vi "Laser.vi"() -> ()   [LabVIEW 2013]
doc: "Пограмма управления мишенью лазерного источника ионов."
uses:
  <vilib>/Utility/miscctls.llb/LVPositionTypeDef.ctl
  <vilib>/Utility/inputDevices.llb/closeJoystick.vi
  <vilib>/Utility/inputDevices.llb/mouseAcquire.vi
panel:
  out "prog ON":string
  out "on event":string
  out "send string":string
  in  "выстрел Y дейт":u16 step=1
  out "Статус":bool=TRUE caption="Готов!"
  in  "Параметры М1":T1={"TipStrip"="Мишень 1", "Left"=1, "Top"=1, "Width"=10, "Height"=10, "Шаг перехода по горизонтали"=3, "Шаг перехода по горизонтали"=3, "Выстрелов до перехода"=10}
  out "Знак Графит Dx":i8=100
  out "Знак LiF2 Dx":i8=100
  out "Знак LiF1 Dx":i8=100
  out "Знак дейт Dx":i8=100
  in  "выстрел  Y Графит":u16 step=1
  in  "выстрел X Графит":u16 step=1
  in  "выстрел Y LiF 2":u16 step=1
  in  "выстрел X LiF 2":u16 step=1
  in  "выстрел Y LiF 1":u16 step=1
  in  "выстрел X LiF 1":u16 step=1
  in  "выстрел X дейт":u16 step=1
  in  "xxx":enum32{" Мишени", " Настройки TCP"}(tab)
  in  "XY лазера":bool
  in  "LiF 1":picture
  in  "Звук выстрела":bool
  in  "Мишень 2":picture
  in  "Мишень 1":picture
  in  "OK Button":bool
  in  "Графит":picture
  in  "Дейтерий":picture
  in  "Выстрелов до перемотки":u16=100
  in  "id мишени":u16=1
  in  "Счетчик выстрелов:":u32
  in  "Шаг перехода по Y графит":dbl=1.0 format="%.1f"
  in  "Шаг перехода по Х графит":dbl=1.0 format="%.1f"
  in  "Выстрелов в точку  графит":u16=3
  in  "Шаг перехода по Y LiF 2":dbl=1.0 format="%.1f"
  in  "Шаг перехода по Х LiF 2":dbl=1.0 format="%.1f"
  in  "Выстрелов в точку  LiF 2":u16=3
  in  "Шаг перехода по Y LiF 1":dbl=1.0 format="%.1f"
  in  "Шаг перехода по Х LiF 1":dbl=1.0 format="%.1f"
  in  "Выстрелов в точку LiF 1":u16=3
  in  "Шаг перехода по Y дейт":dbl=1.0 min=0.0 format="%.1f"
  in  "Шаг перехода по Х дейт":dbl=1.0 min=0.0 format="%.1f"
  in  "Выстрелов в точку дейтерий":u16=3
  in  "TCP read data":string
  in  "LiF 2":picture
  out "Slide X axis":u8(slide) max=100 scale=0.0..100.0
  out "Slide Y axis":u8(slide) max=50 step=1
  in  "Снимок":bool
  out "con err":bool caption="Connect"
  out "Con":bool
  out "Mouse on Pane pos Horizontal":i32
  out "Mouse on Pane pos Vertical":i32
  in  "Выстрел по мишени!":u32
  out "Выбор миш 1":bool
  out "Выбор миш 2":bool
  out "Выбор миш 3":bool
  out "Выбор миш 4":bool
  out "Счетчик мишеней":u16=3
  out "Шаг перехода по горизонтали":u16
  out "Шаг перехода по вертикали":u16
  out "Выстрелов до перехода":u16
  in  "порт":u16=10001
  in  "IP-адрес":string="159.93.126.157"
  in  "Disconnect":bool caption="Disconn"
  out "Connected":bool
  in  "Connect":bool
  out "TCP error source":string
  in  "stop":bool
  out "read_error_indicator":bool
  in  "Connect 2":bool caption="Connect"
  in  "flag1":bool caption="Disconn"
  out "x+1":dbl
  out "TCP con ID":refnum<k5>
  # "LiF 1"
  # "Дейтерированный полиэтилен"
  # "LiF 2"
  # "Графит"
  # "LiF 1"
  # "Графит"
  # "Дейтерированный полиэтилен"
  # "Шаг перехода по Y, мм"
  # "Шаг перехода по Х, мм"
  # "Выстрелов в точку"
  # "Выстрелов в точку"
  # "Шаг перехода по Х, мм"
  # "Шаг перехода по Y, мм"
  # "Выстрелов в точку"
  # "Шаг перехода по Х, мм"
  # "Шаг перехода по Y, мм"
  # "Выстрелов в точку"
  # "Шаг перехода по Х, мм"
  # "Шаг перехода по Y, мм"
  # "LiF 2"
types:
  T1 = cluster{"TipStrip":string, "Left":i32, "Top":i32, "Width":u16, "Height":u16, "Шаг перехода по горизонтали":u16, "Шаг перехода по горизонтали":u16, "Выстрелов до перехода":u16}
  T2 = typedef "LVPositionTypeDef.ctl" = cluster{"Left":i32, "Top":i32}
  T3 = enum8{"Enabled", "Disabled", "Disabled and Grayed Out"}
  T4 = typedef "imagedata.ctl" = cluster{"image type":i32, "image depth":i32, "image":u8[], "mask":u8[], "colors":u32[], "Rectangle":cluster{"left":i16, "top":i16, "right":i16, "bottom":i16}}
  T5 = typedef "LVRectTypeDef.ctl" = cluster{"Left":i16, "Top":i16, "Right":i16, "Bottom":i16}
  T6 = cluster{"Horizontal":i32, "Vertical":i32, "Scrolling":i32}
  T7 = cluster{"Название мишени":string, "Х0":u16, "Y0":u16, "Длина, мм":u16, "Ширина, мм":u16, "Шаг перехода по горизонтали":u16, "Шаг перехода по вертикали":u16, "Выстрелов до перехода":u16}
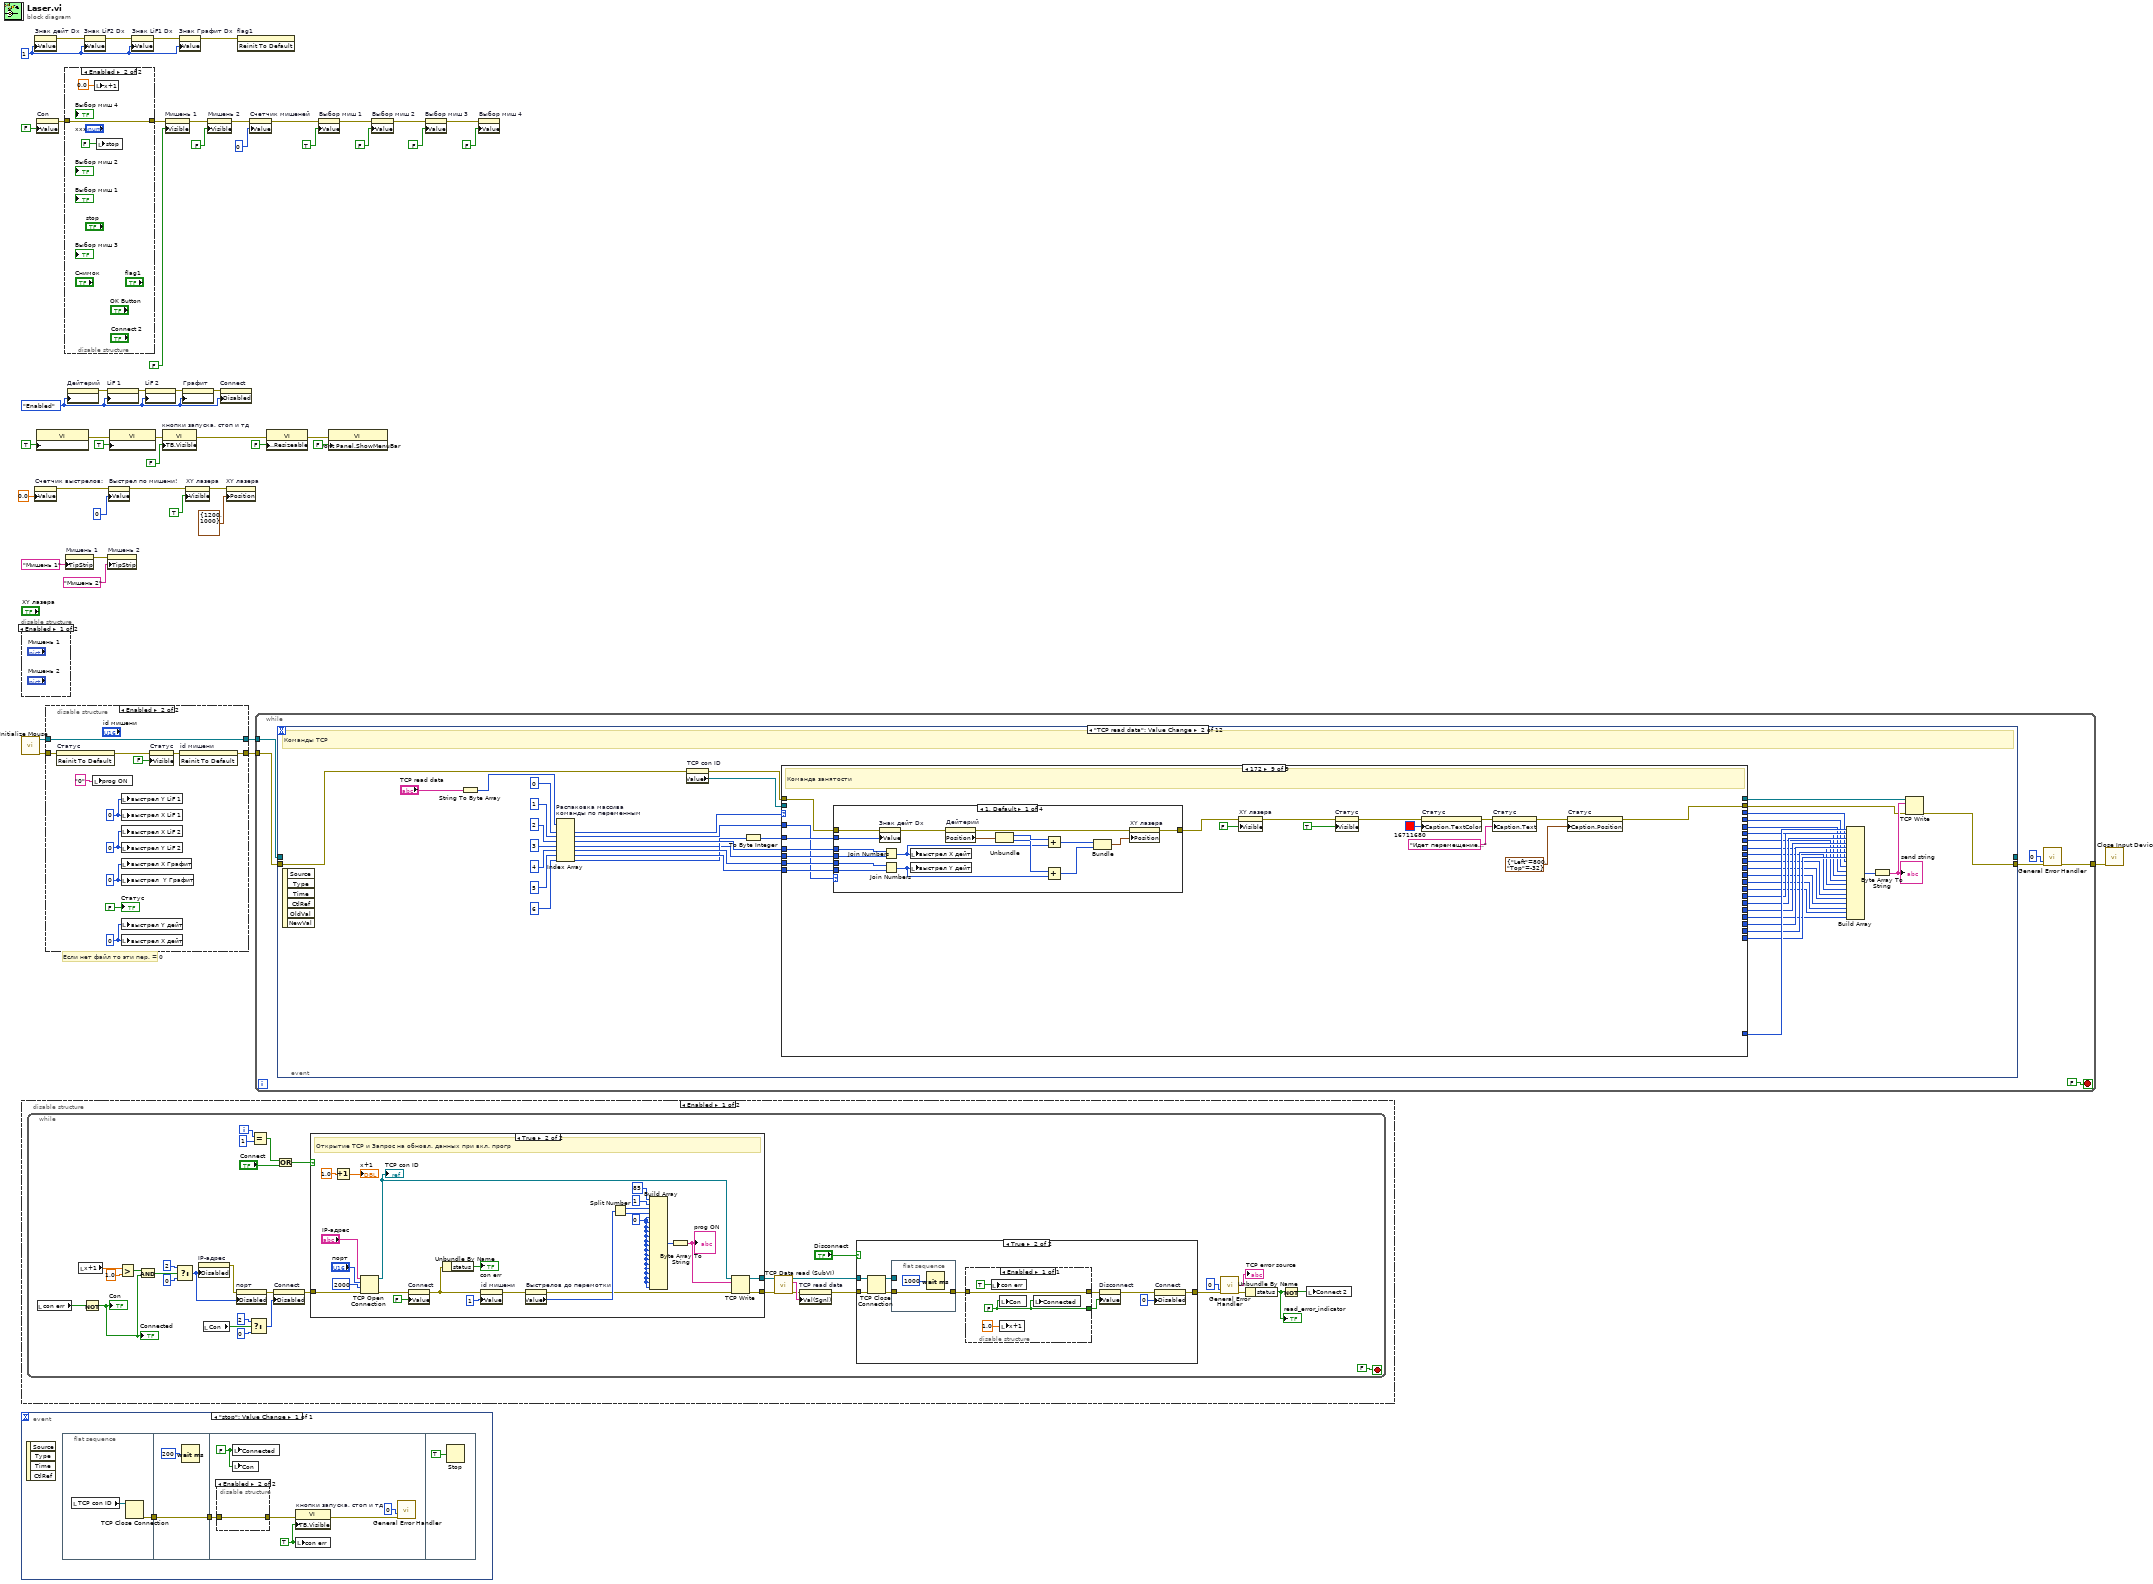
[diagram p0: block diagram]
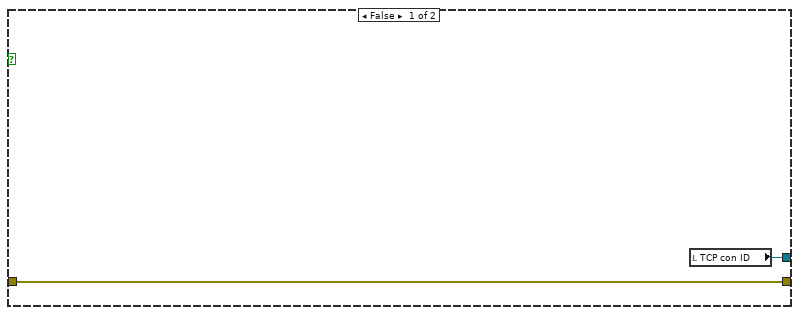
[diagram p3: hidden frame]
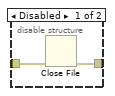
[diagram p8: hidden frame]
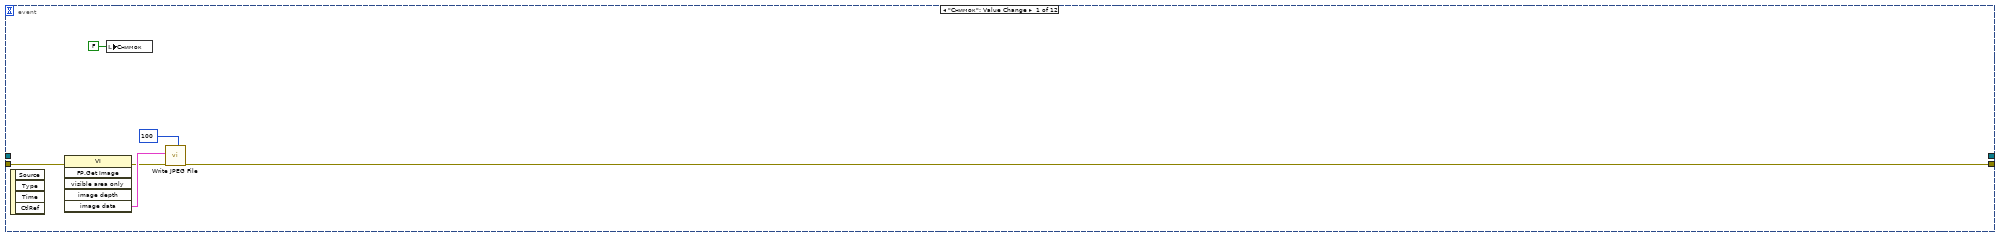
[diagram p9: hidden frame]
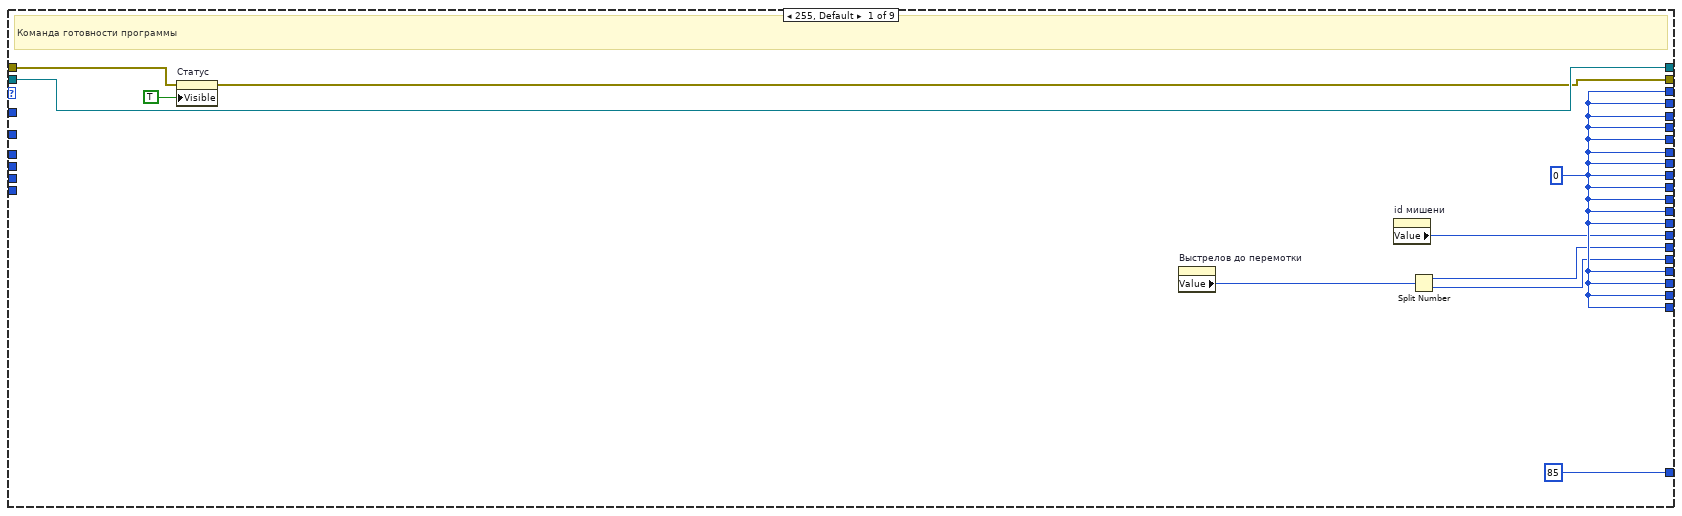
[diagram p10: hidden frame]
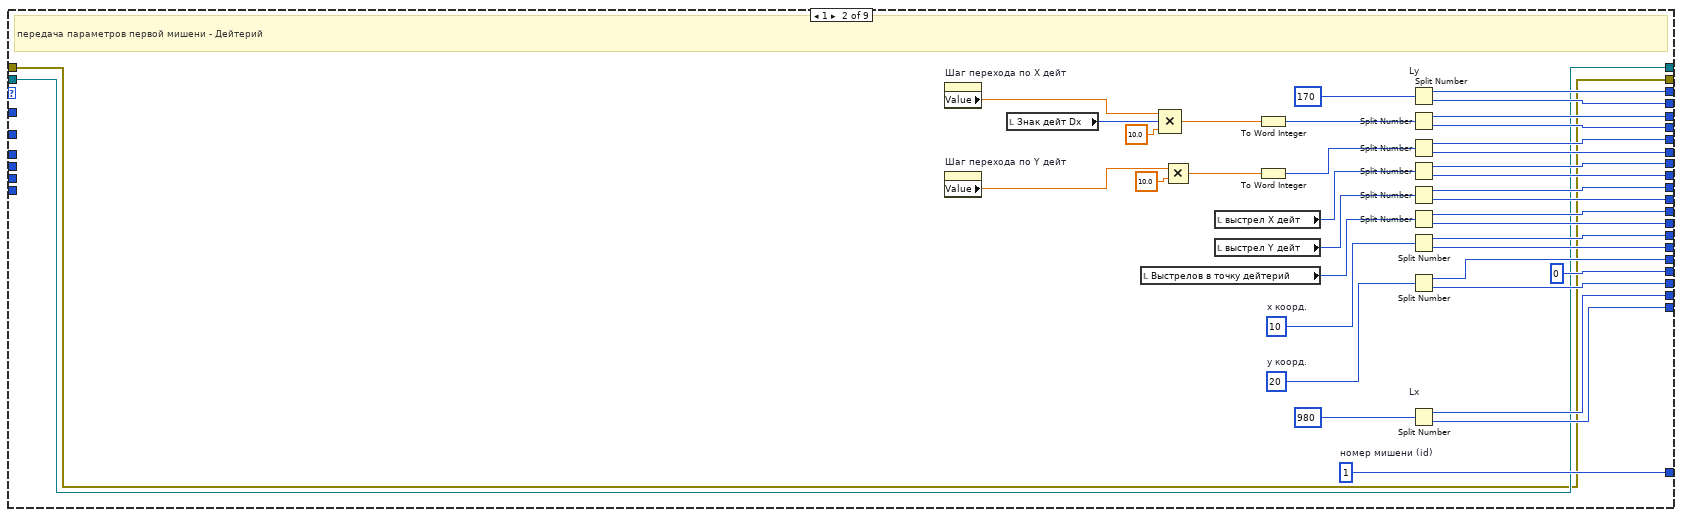
[diagram p11: hidden frame]
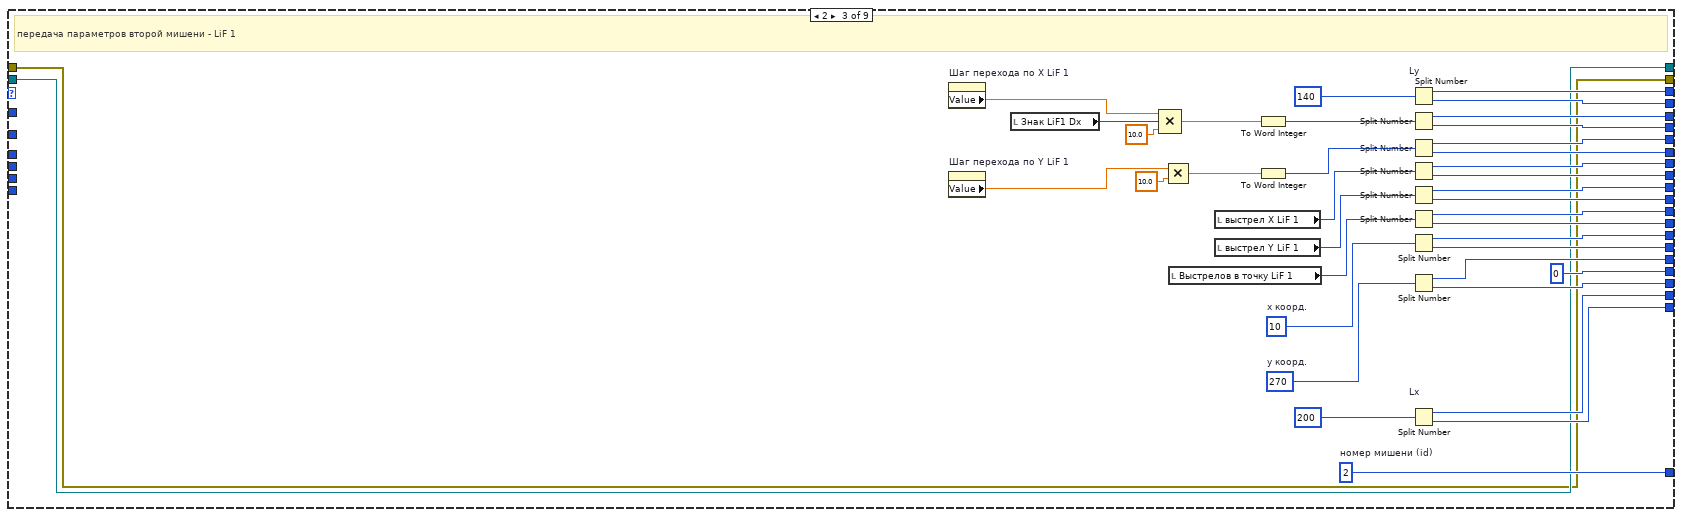
[diagram p12: hidden frame]
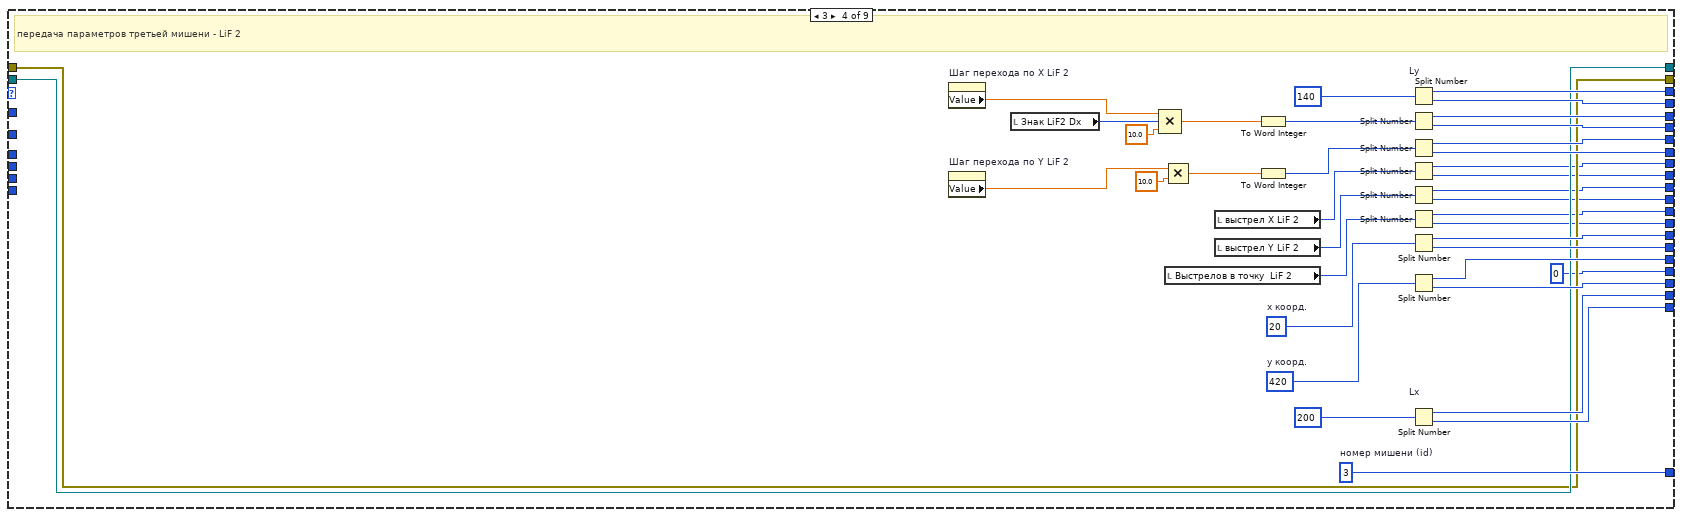
[diagram p13: hidden frame]
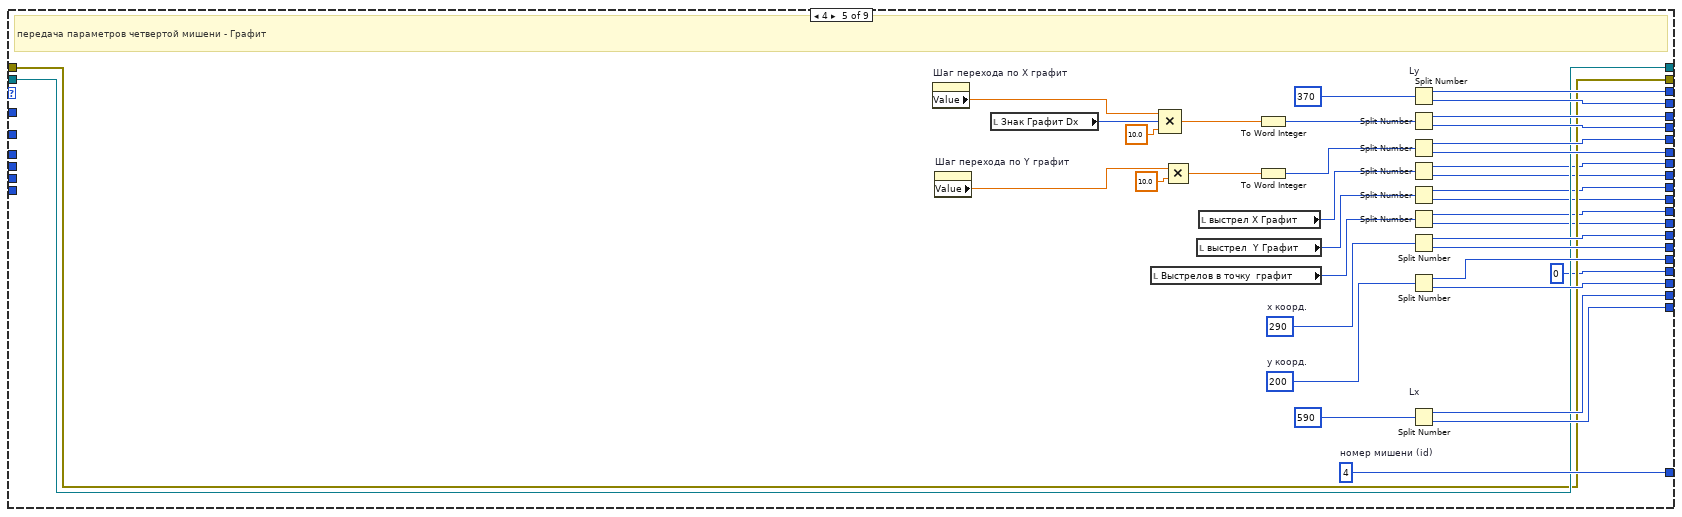
[diagram p14: hidden frame]
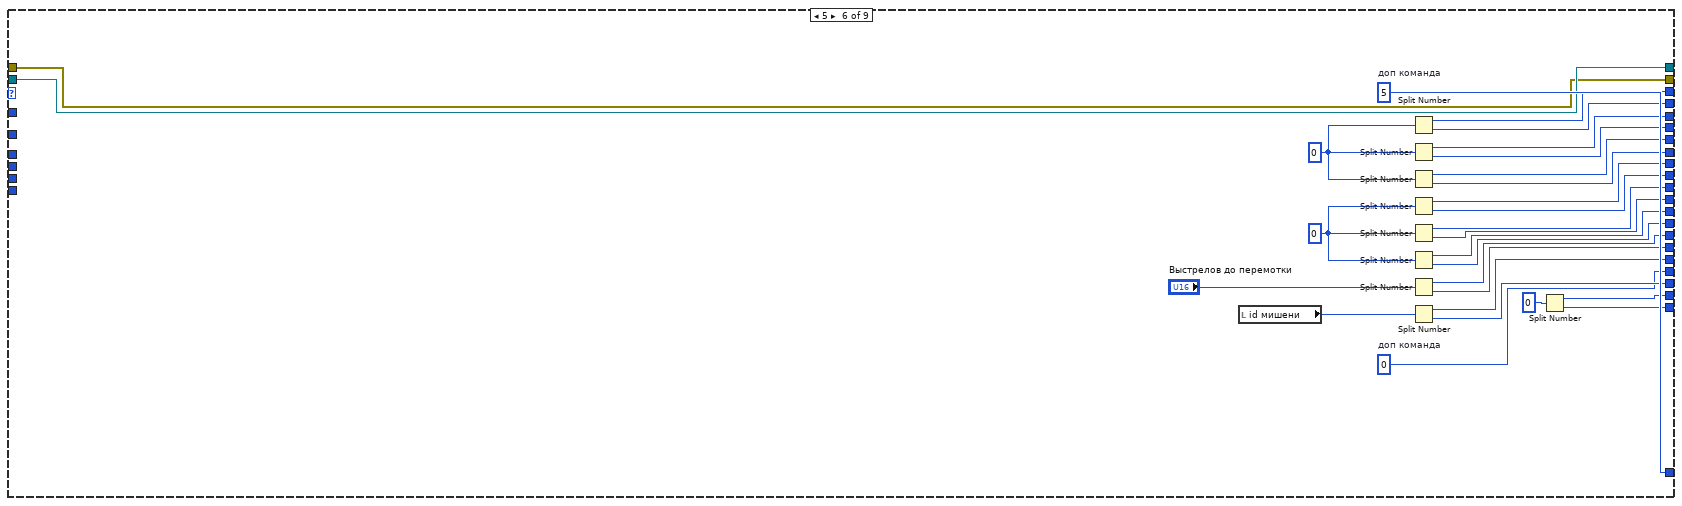
[diagram p15: hidden frame]
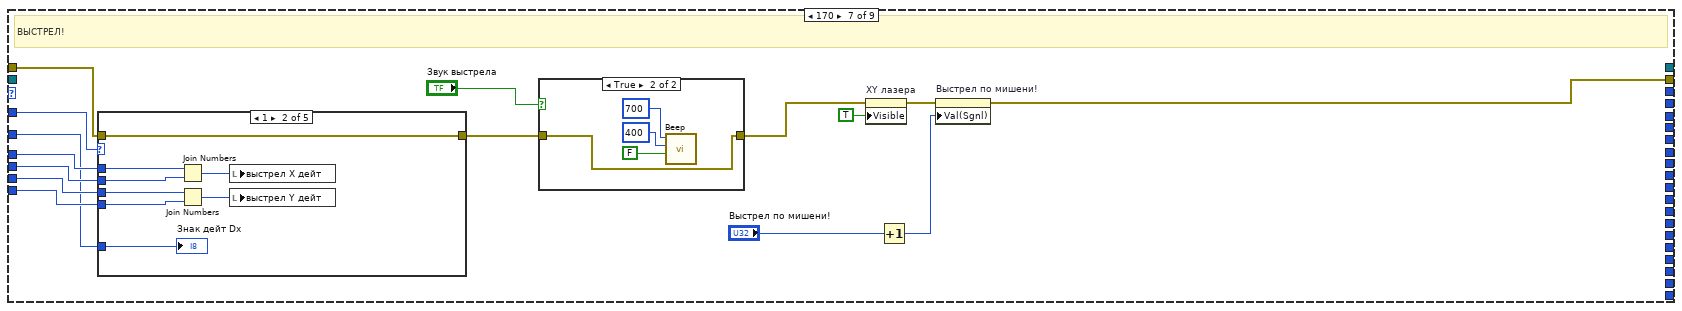
[diagram p16: hidden frame]
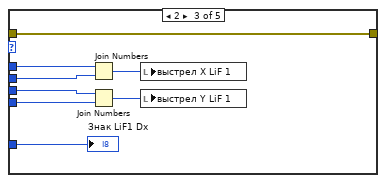
[diagram p19: hidden frame]
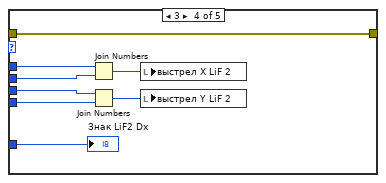
[diagram p20: hidden frame]
diagram:
  w16 = i8 1 ("Знак дейт Dx")
  w2 = T3."Enabled" ("Disabled")
  # "Если нет файл то эти пер. = 0"
  n1 = disable-structure shown="Enabled" {
    frame Enabled {
    }
    frame Disabled {
    }
  }
  n2 = call <vilib>:"Initialize Mouse.vi"() -> ("error out"=w9:errorcluster, "device ID"=w11:refnum<k1>)  [unwired: 1 in, 9 out]
  n3 = disable-structure shown="Enabled" {
    frame Enabled {
      n4 = while {
        i -> [w77]
        stop <- FALSE stop-if-true
        n5 = local read "con err"() -> (w65:bool)
        n6 = local read "x+1"() -> (w68:dbl)
        n7 = Not(x=w65) -> (.not. x?=w64:bool)
        "Connected" <- w64
        "Con" <- w64
        n8 = Greater?(x=w68, y=1.0) -> (0:w66:bool)
        n9 = And(x=w66, y=w64) -> (x .and. y?=w61:bool)
        n10 = Select(t=u8 2 ("Disabled"), s=w61, f=u8 0 ("Disabled")) -> (s? t:f=w83:u8)
        n11 = property on="IP-адрес" class="Str"("Disabled"=w83) -> (error out=w82:errorcluster)  [unwired: 2 in, 1 out]
        n12 = local read "Con"() -> (w58:bool)
        n13 = property on="порт" class="DigNum (strict)"(error in=w82, "Disabled"=w83) -> (error out=w81:errorcluster)  [unwired: 1 in, 1 out]
        n14 = Select(t=u8 2 ("Disabled"), s=w58, f=u8 0 ("Disabled")) -> (s? t:f=w70:u8)
        n15 = Equal?(x=w77, y=1) -> (x = y?=w78:bool)
        n16 = property on="Connect" class="Bool (strict)"(error in=w81, "Disabled"=w70) -> (error out=w75:errorcluster)  [unwired: 1 in, 1 out]
        n17 = Or(x=w78, y="Connect") -> (x .or. y?=w80:bool)
        n18 = case shown="True" w80 {
          tunnel: [w87 w91] -> w55
          tunnel: w75 -> [w87 w103]
          tunnel: [w86 w90] -> w54
          frame False {
            n19 = local read "TCP con ID"() -> (w86:refnum<k5>)
          }
          frame True {
            w98 = u8 0 ("element")
            # "Открытие TCP и Запрос на обновл. данных при вкл. прогр"
            n20 = Increment(x=1.0) -> (x+1=→"x+1":dbl)
            n21 = TCP Open Connection(address="IP-адрес", remote port or service name="порт", timeout ms (60000)=2000, error in (no error)=w103) -> (connection ID=w88:refnum<k5>, error out=w105:errorcluster)  [unwired: 1 out]
            "TCP con ID" <- w88
            n22 = property on="Connect" class="Bool (strict)"(error in=w105, "Value"=FALSE ("Connect")) -> (error out=w93:errorcluster)  [unwired: 1 in, 1 out]
            n23 = Unbundle By Name(w93) -> ("status"=→"con err":bool)
            n24 = property on="id мишени" class="DigNum (strict)"(error in=w93, "Value"=u16 1 ("id мишени")) -> (error out=w95:errorcluster)  [unwired: 1 in, 1 out]
            n25 = property on="Выстрелов до перемотки" class="DigNum (strict)"(error in=w95) -> (error out=w92:errorcluster, "Value"=w99:u16)  [unwired: 1 in, 1 out]
            n26 = Split Number(x=w99) -> (hi(x)=w97:u8, lo(x)=w96:u8)
            n27 = Build Array(u8 85 ("element"), u16 1 ("id мишени"), w97, w96, w98, w98, w98, w98, w98, w98, w98, w98, w98, w98, w98, w98, w98, w98, w98, w98) -> (w101:u16[])
            n28 = Byte Array To String(unsigned byte array=w101) -> (string=w100:string)
            "prog ON" <- w100
            n29 = TCP Write(connection ID=w88, data in=w100, error in (no error)=w92) -> (connection ID out=w90:refnum<k5>, error out=w91:errorcluster)  [unwired: 1 in, 1 out]
          }
        }
        n30 = call "TCP Data read (SubVI).vi"("error in (no error)"=w55, "TCP Network Connection in"=w54) -> ("error out"=w56:errorcluster, "Read data"=w71:string, "TCP Network Connection out"=w73:refnum<k5>)  [unwired: 1 in, 6 out]
        n31 = property on="TCP read data" class="Str"(error in=w56, "Val(Sgnl)"=w71) -> (error out=w57:errorcluster)  [unwired: 1 in, 1 out]
        n32 = case shown="True" "Disconnect" {
          tunnel: [w112 w118] -> w52
          tunnel: w57 -> [w112 w117]
          tunnel: w73 -> [_ w116]
          frame False {
          }
          frame True {
            n33 = TCP Close Connection(connection ID=w116, error in (no error)=w117) -> (connection ID out=w120:refnum<k5>, error out=w119:errorcluster)  [unwired: 1 out]
            n34 = flat-sequence {
              tunnel: w120 -> [_]
              tunnel: w119 -> [w127]
              tunnel: [w127] -> w113
              frame #0 {
                n35 = Wait (ms)(milliseconds to wait=u32 1000) -> ()  [unwired: 1 out]
              }
            }
            n36 = disable-structure shown="Enabled" {
              disable-tunnel: [w124] -> w115
              disable-tunnel: [w123] -> w114
              disable-tunnel: w113 -> [w123]
              frame Enabled {
                w124 = FALSE ("Disconnect")
                n37 = local write "con err"(TRUE ("con err")) -> ()
                n38 = local write "Con"(w124) -> ()
                n39 = local write "x+1"(1.0 ("1")) -> ()
                n40 = local write "Connected"(w124) -> ()
              }
            }
            n41 = property on="Disconnect" class="Bool (strict)"(error in=w114, "Value"=w115) -> (error out=w121:errorcluster)  [unwired: 1 in, 1 out]
            n42 = property on="Connect" class="Bool (strict)"(error in=w121, "Disabled"=u8 0) -> (error out=w118:errorcluster)  [unwired: 1 in, 1 out]
          }
        }
        n43 = call <vilib>:"General Error Handler.vi"("type of dialog (OK msg:1)"=u8 0, "error in (no error)"=w52) -> ("source out"=→"TCP error source":string, "error out"=w51:errorcluster)  [unwired: 12 out]
        n44 = Unbundle By Name(w51) -> ("status"=w53:bool)
        "read_error_indicator" <- w53
        n45 = Not(x=w53) -> (.not. x?=w85:bool)
        n46 = local write "Connect 2"(w85) -> ()
      }
    }
    frame Disabled {
    }
  }
  n47 = event shown="[0] \"stop\": Value Change" {
    selector: _ -> [_]
    dyn-events: _ -> [_]
    timeout: _ -> [_]
    event "stop": Value Change {
      n48 = event-data() -> ()  [unwired: 5 out]
      n49 = flat-sequence {
        tunnel: [w131] -> w130
        tunnel: w130 -> [w134]
        tunnel: [w134] -> w129
        tunnel: w129 -> [w138]
        frame #0 {
          n50 = local read "TCP con ID"() -> (w132:refnum<k5>)
          n51 = TCP Close Connection(connection ID=w132) -> (error out=w131:errorcluster)  [unwired: 1 in, 2 out]
        }
        frame #1 {
          n52 = Wait (ms)(milliseconds to wait=u32 200) -> ()  [unwired: 1 out]
        }
        frame #2 {
          w140 = FALSE ("Запись в файл")
          w139 = TRUE ("Tool Bar:Visible")
          n53 = disable-structure shown="Enabled" {
            disable-tunnel: [w142 w143] -> w136
            disable-tunnel: w138 -> [w141 w143]
            frame Disabled {
              n54 = Close File(error in=w141) -> (error out=w142:errorcluster)  [unwired: 1 in, 1 out]
            }
            frame Enabled {
            }
          }
          n55 = local write "Connected"(w140) -> ()
          n56 = local write "Con"(w140) -> ()
          n57 = property on="кнопки запуска, стоп и тд" class="VI"(error in=w136, "TB.Visible"=w139) -> (error out=w137:errorcluster)  [unwired: 1 in, 1 out]
          n58 = local write "con err"(w139) -> ()
          n59 = call <vilib>:"General Error Handler.vi"("type of dialog (OK msg:1)"=u32 0 ("milliseconds to wait"), "error in (no error)"=w137) -> ()  [unwired: 14 out]
        }
        frame #3 {
          n60 = Stop(stop? (T)=TRUE) -> ()
        }
      }
    }
  }
  n61 = property on="Знак дейт Dx" class="DigNum (strict)"("Value"=w16) -> (error out=w15:errorcluster)  [unwired: 2 in, 1 out]
  n62 = property on="Счетчик выстрелов:" class="DigNum (strict)"("Value"=0.0 ("Счетчик выстрелов:")) -> (error out=w32:errorcluster)  [unwired: 2 in, 1 out]
  n63 = property on="Con" class="Bool (strict)"("Value"=FALSE ("Connected")) -> (error out=w38:errorcluster)  [unwired: 2 in, 1 out]
  n64 = property class="VI"("Front Panel.Minimizeable"=TRUE ("Front Panel Window:Minimizable")) -> (error out=w44:errorcluster)  [unwired: 2 in, 1 out]
  n65 = disable-structure shown="Enabled" {
    disable-tunnel: [_ w152] -> w12
    disable-tunnel: w11 -> [_ w152]
    disable-tunnel: [_ w147] -> w10
    disable-tunnel: w9 -> [_ w150]
    frame Disabled {
    }
    frame Enabled {
      w153 = u16 0 ("выстрел  Y Графит")
      w154 = u16 0 ("выстрел Y LiF 2")
      w155 = u16 0 ("выстрел X LiF 1")
      w156 = u16 0 ("выстрел X дейт")
      n66 = invoke on="Статус" class="Bool (strict)" method="Reinit To Default"(error in=w150) -> (error out=w148:errorcluster)  [unwired: 2 in, 2 out]
      n67 = local write "prog ON"("0" ("prog ON")) -> ()
      n68 = local write "выстрел Y LiF 1"(w155) -> ()
      n69 = local write "выстрел X LiF 1"(w155) -> ()
      n70 = local write "выстрел X LiF 2"(w154) -> ()
      n71 = local write "выстрел Y LiF 2"(w154) -> ()
      n72 = local write "выстрел X Графит"(w153) -> ()
      n73 = local write "выстрел  Y Графит"(w153) -> ()
      n74 = local write "выстрел Y дейт"(w156) -> ()
      n75 = local write "выстрел X дейт"(w156) -> ()
      n76 = property on="Статус" class="Bool (strict)"(error in=w148, "Visible"=FALSE) -> (error out=w146:errorcluster)  [unwired: 1 in, 1 out]
      n77 = invoke on="id мишени" class="DigNum (strict)" method="Reinit To Default"(error in=w146) -> (error out=w147:errorcluster)  [unwired: 2 in, 2 out]
      "Статус" <- FALSE ("Готов")
    }
  }
  n78 = disable-structure shown="Enabled" {
    disable-tunnel: [_ w157] -> w3
    disable-tunnel: w38 -> [_ w157]
    frame Disabled {
    }
    frame Enabled {
      n79 = local write "x+1"(0.0 ("x+1")) -> ()
      n80 = local write "stop"(FALSE ("Boolean")) -> ()
    }
  }
  n81 = property on="Мишень 1" class="Pict"("TipStrip"="Мишень 1" ("Tip Strip")) -> (error out=w6:errorcluster)  [unwired: 2 in, 1 out]
  n82 = property on="Дейтерий" class="Pict"("DisabledEnum"=w2) -> (error out=w22:errorcluster)  [unwired: 2 in, 1 out]
  n83 = property on="Знак LiF2 Dx" class="DigNum (strict)"(error in=w15, "Value"=w16) -> (error out=w14:errorcluster)  [unwired: 1 in, 1 out]
  n84 = property on="LiF 1" class="Pict"(error in=w22, "DisabledEnum"=w2) -> (error out=w21:errorcluster)  [unwired: 1 in, 1 out]
  n85 = property on="Мишень 2" class="Pict"(error in=w6, "TipStrip"="Мишень 2" ("Tip Strip")) -> ()  [unwired: 1 in, 2 out]
  n86 = property on="Выстрел по мишени!" class="DigNum (strict)"(error in=w32, "Value"=u32 0 ("Выстрел по мишени!")) -> (error out=w19:errorcluster)  [unwired: 1 in, 1 out]
  n87 = property class="VI"(error in=w44, "Front Panel.TitleBarVis"=TRUE ("Front Panel Window:Title Bar Visible")) -> (error out=w43:errorcluster)  [unwired: 1 in, 1 out]
  n88 = property on="Знак LiF1 Dx" class="DigNum (strict)"(error in=w14, "Value"=w16) -> (error out=w13:errorcluster)  [unwired: 1 in, 1 out]
  n89 = property on="LiF 2" class="Pict"(error in=w21, "DisabledEnum"=w2) -> (error out=w20:errorcluster)  [unwired: 1 in, 1 out]
  n90 = property on="кнопки запуска, стоп и тд" class="VI"(error in=w43, "TB.Visible"=FALSE ("Tool Bar:Visible")) -> (error out=w42:errorcluster)  [unwired: 1 in, 1 out]
  n91 = property on="Мишень 1" class="Pict"(error in=w3, "Visible"=FALSE) -> (error out=w36:errorcluster)  [unwired: 1 in, 1 out]
  n92 = property on="Знак Графит Dx" class="DigNum (strict)"(error in=w13, "Value"=w16) -> (error out=w5:errorcluster)  [unwired: 1 in, 1 out]
  n93 = property on="Графит" class="Pict"(error in=w20, "DisabledEnum"=w2) -> (error out=w4:errorcluster)  [unwired: 1 in, 1 out]
  n94 = property on="XY лазера" class="Bool (strict)"(error in=w19, "Visible"=TRUE) -> (error out=w17:errorcluster)  [unwired: 1 in, 1 out]
  n95 = property on="Мишень 2" class="Pict"(error in=w36, "Visible"=FALSE) -> (error out=w33:errorcluster)  [unwired: 1 in, 1 out]
  n96 = property on="Connect" class="Bool (strict)"(error in=w4, "Disabled"=w2) -> ()  [unwired: 1 in, 2 out]
  n97 = property on="XY лазера" class="Bool (strict)"(error in=w17, "Position"=T2 {"Left"=1200, "Top"=1000}) -> ()  [unwired: 1 in, 2 out]
  n98 = invoke on="flag1" class="Bool (strict)" method="Reinit To Default"(error in=w5) -> ()  [unwired: 2 in, 3 out]
  n99 = property on="Счетчик мишеней" class="DigNum (strict)"(error in=w33, "Value"=u16 0 ("Счетчик мишеней")) -> (error out=w24:errorcluster)  [unwired: 1 in, 1 out]
  n100 = while {
    tunnel: w10 -> [w164]
    tunnel: w12 -> [w163]
    tunnel: [w160] -> w1
    stop <- FALSE stop-if-true
    n101 = event shown="[1] \"TCP read data\": Value Change" {
      selector: _ -> [_ _ _ _ _ _ _ _ _ _ _ _]
      dyn-events: _ -> [_ _ _ _ _ _ _ _ _ _ _ _]
      timeout: _ -> [_ _ _ _ _ _ _ _ _ _ _ _]
      tunnel: [w167 w187 w646 w706 w741 w773 w805 w867 w878 w893 w918 _] -> w161
      tunnel: w164 -> [w166 w215 w633 w708 w742 w774 w806 w847 w877 w894 w919 _]
      tunnel: w163 -> [_ _ _ _ _ _ _ w874 _ _ _ _]
      tunnel: [_ _ _ _ _ _ _ w873 _ _ _ _] -> _
      event "Снимок": Value Change {
        n102 = event-data() -> ()  [unwired: 5 out]
        n103 = invoke class="VI" method="FP.Get Image"(error in=w166) -> (error out=w168:errorcluster, "image data"=w169:T4)  [unwired: 5 in, 4 out]
        n104 = local write "Снимок"(FALSE ("Снимок")) -> ()
        n105 = call <vilib>:"Write JPEG File.vi"("quality (80)"=100, "error in (no error)"=w168, "image data"=w169) -> ("error out"=w167:errorcluster)  [unwired: 1 in, 7 out]
      }
      event "TCP read data": Value Change {
        # "Команды TCP"
        n106 = event-data() -> ()  [unwired: 7 out]
        n107 = String To Byte Array(string="TCP read data") -> (unsigned byte array=w180:u8[])
        n108 = Index Array "Распаковка массива\nкоманды по переменным"(array=w180, index #1=0 ("index"), index #2=1 ("index"), index #3=2 ("index"), index #4=3 ("index"), index #5=4 ("index"), index #6=5 ("index"), index #7=6 ("index")) -> (element #1=w212:u8, element #2=w186:u8, element #3=w185:u8, element #4=w172:u8, element #5=w184:u8, element #6=w183:u8, element #7=w182:u8)
        n109 = property on="TCP con ID" class="Ref (strict)"(error in=w215) -> (error out=w214:errorcluster, "Value"=w213:refnum<k5>)  [unwired: 1 in, 1 out]
        n110 = To Byte Integer(number=w182) -> (8bit integer=w181:i8)
        n111 = case shown="172" w212 {
          tunnel: w214 -> [w218 w231 w269 w317 w355 w381 w410 w469 w550]
          tunnel: w213 -> [w225 w232 w270 w318 w356 w392 _ _ _]
          tunnel: [u8 85 ("доп команда") w252 w290 w340 w378 w405 _ _ _] -> w209
          tunnel: [w223 w251 w289 w338 w376 w404 _ _ _] -> w208
          tunnel: [w221 w250 w288 w337 w375 w403 _ _ _] -> w207
          tunnel: [w220 w249 w287 w328 w366 w402 _ _ _] -> w206
          tunnel: [w224 w248 w286 w327 w365 w401 _ _ _] -> w205
          tunnel: [w224 w247 w285 w326 w364 w400 _ _ _] -> w204
          tunnel: [w224 w246 w284 w325 w363 w399 _ _ _] -> w203
          tunnel: [w224 w245 w283 w324 w362 w398 _ _ _] -> w202
          tunnel: [w224 w244 w282 w323 w361 w397 _ _ _] -> w201
          tunnel: [w224 w243 w281 w322 w360 w396 _ _ _] -> w200
          tunnel: [w224 w242 w280 w321 w359 w395 _ _ _] -> w199
          tunnel: [w224 w240 w279 w320 w358 w394 _ _ _] -> w198
          tunnel: [w224 w239 w278 w319 w357 w393 _ _ _] -> w197
          tunnel: [w224 u8 0 u8 0 u8 0 ("номер мишени (id)") u8 0 ("номер мишени (id)") w387 _ _ _] -> w196
          tunnel: [w224 w238 w276 w315 w353 w391 _ _ _] -> w195
          tunnel: [w224 w237 w275 w314 w352 w390 _ _ _] -> w194
          tunnel: [w224 w236 w274 w312 w350 w389 _ _ _] -> w193
          tunnel: [w224 w235 w273 w311 w349 w388 _ _ _] -> w192
          tunnel: [w224 w234 w272 w308 w346 w386 _ _ _] -> w191
          tunnel: [w224 w233 w271 w307 w345 w385 _ _ _] -> w190
          tunnel: [w225 w232 w270 w318 w356 w392 _ _ _] -> w189
          tunnel: [w217 w231 w269 w317 w355 w381 w406 w461 w552] -> w188
          tunnel: w186 -> [_ _ _ _ _ _ w416 w474 w543]
          tunnel: w185 -> [_ _ _ _ _ _ w420 w470 w547]
          tunnel: w172 -> [_ _ _ _ _ _ w419 w471 w546]
          tunnel: w184 -> [_ _ _ _ _ _ w418 w472 w545]
          tunnel: w183 -> [_ _ _ _ _ _ w417 w473 w544]
          tunnel: w181 -> [_ _ _ _ _ _ w411 w465 w548]
          frame 255, Default {
            w224 = u8 0
            # "Команда готовности программы"
            n112 = property on="Статус" class="Bool (strict)"(error in=w218, "Visible"=TRUE) -> (error out=w217:errorcluster)  [unwired: 1 in, 1 out]
            n113 = property on="Выстрелов до перемотки" class="DigNum (strict)"() -> ("Value"=w222:u16)  [unwired: 2 in, 2 out]
            n114 = property on="id мишени" class="DigNum (strict)"() -> ("Value"=w223:u16)  [unwired: 2 in, 2 out]
            n115 = Split Number(x=w222) -> (hi(x)=w221:u8, lo(x)=w220:u8)
          }
          frame 1 {
            w252 = u8 1  # номер мишени (id)
            w260 = u16 20  # y коорд.
            w261 = u16 10  # x коорд.
            # "передача параметров первой мишени - Дейтерий"
            n116 = property on="Шаг перехода по Х дейт" class="DigNum (strict)"() -> ("Value"=w227:dbl)  [unwired: 2 in, 2 out]
            n117 = property on="Шаг перехода по Y дейт" class="DigNum (strict)"() -> ("Value"=w263:dbl)  [unwired: 2 in, 2 out]
            n118 = local read "Знак дейт Dx"() -> (w229:i8)
            n119 = local read "Выстрелов в точку дейтерий"() -> (w253:u16)
            n120 = Compound Arithmetic op=MULTIPLY(w227, w229, 10.0 ("y")) -> (w228:dbl)
            n121 = Multiply(x=w263, y=10.0) -> (x*y=w262:dbl)
            n122 = local read "выстрел X дейт"() -> (w255:u16)
            n123 = local read "выстрел Y дейт"() -> (w254:u16)
            n124 = To Word Integer(number=w228) -> (16bit integer=w257:i16)
            n125 = To Word Integer(number=w262) -> (16bit integer=w256:i16)
            n126 = Split Number "Ly"(x=u16 170) -> (hi(x)=w245:u8, lo(x)=w244:u8)
            n127 = Split Number(x=w257) -> (hi(x)=w243:u8, lo(x)=w242:u8)
            n128 = Split Number(x=w256) -> (hi(x)=w240:u8, lo(x)=w239:u8)
            n129 = Split Number(x=w255) -> (hi(x)=w238:u8, lo(x)=w237:u8)
            n130 = Split Number(x=w254) -> (hi(x)=w236:u8, lo(x)=w235:u8)
            n131 = Split Number(x=w253) -> (hi(x)=w234:u8, lo(x)=w233:u8)
            n132 = Split Number(x=w261) -> (hi(x)=w251:u8, lo(x)=w250:u8)
            n133 = Split Number(x=w260) -> (hi(x)=w249:u8, lo(x)=w248:u8)
            n134 = Split Number "Lx"(x=u16 980) -> (hi(x)=w247:u8, lo(x)=w246:u8)
          }
          frame 2 {
            w290 = u8 2  # номер мишени (id)
            w301 = u16 270  # y коорд.
            w302 = u16 10  # x коорд.
            # "передача параметров второй мишени - LiF 1"
            n135 = property on="Шаг перехода по Х LiF 1" class="DigNum (strict)"() -> ("Value"=w268:dbl)  [unwired: 2 in, 2 out]
            n136 = property on="Шаг перехода по Y LiF 1" class="DigNum (strict)"() -> ("Value"=w296:dbl)  [unwired: 2 in, 2 out]
            n137 = local read "Знак LiF1 Dx"() -> (w265:i8)
            n138 = Compound Arithmetic op=MULTIPLY(w268, w265, 10.0 ("y")) -> (w266:dbl)
            n139 = Multiply(x=w296, y=10.0) -> (x*y=w297:dbl)
            n140 = local read "Выстрелов в точку LiF 1"() -> (w291:u16)
            n141 = local read "выстрел X LiF 1"() -> (w293:u16)
            n142 = local read "выстрел Y LiF 1"() -> (w292:u16)
            n143 = To Word Integer(number=w266) -> (16bit integer=w295:i16)
            n144 = To Word Integer(number=w297) -> (16bit integer=w294:i16)
            n145 = Split Number "Ly"(x=u16 140) -> (hi(x)=w283:u8, lo(x)=w282:u8)
            n146 = Split Number(x=w295) -> (hi(x)=w281:u8, lo(x)=w280:u8)
            n147 = Split Number(x=w294) -> (hi(x)=w279:u8, lo(x)=w278:u8)
            n148 = Split Number(x=w293) -> (hi(x)=w276:u8, lo(x)=w275:u8)
            n149 = Split Number(x=w292) -> (hi(x)=w274:u8, lo(x)=w273:u8)
            n150 = Split Number(x=w291) -> (hi(x)=w272:u8, lo(x)=w271:u8)
            n151 = Split Number(x=w302) -> (hi(x)=w289:u8, lo(x)=w288:u8)
            n152 = Split Number(x=w301) -> (hi(x)=w287:u8, lo(x)=w286:u8)
            n153 = Split Number "Lx"(x=u16 200) -> (hi(x)=w285:u8, lo(x)=w284:u8)
          }
          frame 3 {
            w333 = u16 420  # y коорд.
            w339 = u16 20  # x коорд.
            w340 = u8 3  # номер мишени (id)
            # "передача параметров третьей мишени - LiF 2"
            n154 = property on="Шаг перехода по Х LiF 2" class="DigNum (strict)"() -> ("Value"=w304:dbl)  [unwired: 2 in, 2 out]
            n155 = property on="Шаг перехода по Y LiF 2" class="DigNum (strict)"() -> ("Value"=w336:dbl)  [unwired: 2 in, 2 out]
            n156 = local read "Знак LiF2 Dx"() -> (w305:i8)
            n157 = Compound Arithmetic op=MULTIPLY(w304, w305, 10.0 ("y")) -> (w303:dbl)
            n158 = Multiply(x=w336, y=10.0) -> (x*y=w334:dbl)
            n159 = local read "Выстрелов в точку  LiF 2"() -> (w309:u16)
            n160 = local read "выстрел X LiF 2"() -> (w316:u16)
            n161 = local read "выстрел Y LiF 2"() -> (w313:u16)
            n162 = To Word Integer(number=w303) -> (16bit integer=w330:i16)
            n163 = To Word Integer(number=w334) -> (16bit integer=w329:i16)
            n164 = Split Number "Ly"(x=u16 140) -> (hi(x)=w324:u8, lo(x)=w323:u8)
            n165 = Split Number(x=w330) -> (hi(x)=w322:u8, lo(x)=w321:u8)
            n166 = Split Number(x=w329) -> (hi(x)=w320:u8, lo(x)=w319:u8)
            n167 = Split Number(x=w316) -> (hi(x)=w315:u8, lo(x)=w314:u8)
            n168 = Split Number(x=w313) -> (hi(x)=w312:u8, lo(x)=w311:u8)
            n169 = Split Number(x=w309) -> (hi(x)=w308:u8, lo(x)=w307:u8)
            n170 = Split Number(x=w339) -> (hi(x)=w338:u8, lo(x)=w337:u8)
            n171 = Split Number(x=w333) -> (hi(x)=w328:u8, lo(x)=w327:u8)
            n172 = Split Number "Lx"(x=u16 200) -> (hi(x)=w326:u8, lo(x)=w325:u8)
          }
          frame 4 {
            w371 = u16 200  # y коорд.
            w377 = u16 290  # x коорд.
            w378 = u8 4  # номер мишени (id)
            # "передача параметров четвертой мишени - Графит"
            n173 = property on="Шаг перехода по Х графит" class="DigNum (strict)"() -> ("Value"=w342:dbl)  [unwired: 2 in, 2 out]
            n174 = property on="Шаг перехода по Y графит" class="DigNum (strict)"() -> ("Value"=w374:dbl)  [unwired: 2 in, 2 out]
            n175 = local read "Знак Графит Dx"() -> (w343:i8)
            n176 = local read "Выстрелов в точку  графит"() -> (w347:u16)
            n177 = Compound Arithmetic op=MULTIPLY(w342, w343, 10.0 ("y")) -> (w341:dbl)
            n178 = Multiply(x=w374, y=10.0) -> (x*y=w372:dbl)
            n179 = local read "выстрел  Y Графит"() -> (w351:u16)
            n180 = local read "выстрел X Графит"() -> (w354:u16)
            n181 = To Word Integer(number=w341) -> (16bit integer=w368:i16)
            n182 = To Word Integer(number=w372) -> (16bit integer=w367:i16)
            n183 = Split Number "Ly"(x=u16 370) -> (hi(x)=w362:u8, lo(x)=w361:u8)
            n184 = Split Number(x=w368) -> (hi(x)=w360:u8, lo(x)=w359:u8)
            n185 = Split Number(x=w367) -> (hi(x)=w358:u8, lo(x)=w357:u8)
            n186 = Split Number(x=w354) -> (hi(x)=w353:u8, lo(x)=w352:u8)
            n187 = Split Number(x=w351) -> (hi(x)=w350:u8, lo(x)=w349:u8)
            n188 = Split Number(x=w347) -> (hi(x)=w346:u8, lo(x)=w345:u8)
            n189 = Split Number(x=w377) -> (hi(x)=w376:u8, lo(x)=w375:u8)
            n190 = Split Number(x=w371) -> (hi(x)=w366:u8, lo(x)=w365:u8)
            n191 = Split Number "Lx"(x=u16 590) -> (hi(x)=w364:u8, lo(x)=w363:u8)
          }
          frame 5 {
            w379 = u16 0
            w383 = u16 0
            w387 = u8 0  # доп команда
            w405 = u8 5  # доп команда
            n192 = local read "id мишени"() -> (w382:u16)
            n193 = Split Number ("Ly")(x=w379) -> (hi(x)=w398:u8, lo(x)=w397:u8)
            n194 = Split Number(x=w379) -> (hi(x)=w396:u8, lo(x)=w395:u8)
            n195 = Split Number(x=w379) -> (hi(x)=w394:u8, lo(x)=w393:u8)
            n196 = Split Number(x=w383) -> (hi(x)=w391:u8, lo(x)=w390:u8)
            n197 = Split Number(x=w383) -> (hi(x)=w389:u8, lo(x)=w388:u8)
            n198 = Split Number(x=w383) -> (hi(x)=w386:u8, lo(x)=w385:u8)
            n199 = Split Number(x="Выстрелов до перемотки") -> (hi(x)=w404:u8, lo(x)=w403:u8)
            n200 = Split Number(x=w382) -> (hi(x)=w402:u8, lo(x)=w401:u8)
            n201 = Split Number ("Lx")(x=u16 0) -> (hi(x)=w400:u8, lo(x)=w399:u8)
          }
          frame 170 {
            # "ВЫСТРЕЛ!"
            n202 = case shown="1" w416 {
              tunnel: w420 -> [_ w434 w442 w450 w458]
              tunnel: w419 -> [_ w433 w441 w449 w457]
              tunnel: w418 -> [_ w431 w439 w447 w455]
              tunnel: w417 -> [_ w430 w438 w446 w454]
              tunnel: w411 -> [_ w427 w436 w443 w452]
              tunnel: [w426 w428 w435 w444 w451] -> w408
              tunnel: w410 -> [w426 w428 w435 w444 w451]
              frame 0, Default {
              }
              frame 1 {
                n203 = Join Numbers(hi=w434, lo=w433) -> ((hi.lo)=w432:u16)
                n204 = Join Numbers(hi=w431, lo=w430) -> ((hi.lo)=w429:u16)
                n205 = local write "выстрел X дейт"(w432) -> ()
                n206 = local write "выстрел Y дейт"(w429) -> ()
                "Знак дейт Dx" <- w427
              }
              frame 2 {
                n207 = Join Numbers(hi=w442, lo=w441) -> ((hi.lo)=w440:u16)
                n208 = Join Numbers(hi=w439, lo=w438) -> ((hi.lo)=w437:u16)
                n209 = local write "выстрел X LiF 1"(w440) -> ()
                n210 = local write "выстрел Y LiF 1"(w437) -> ()
                "Знак LiF1 Dx" <- w436
              }
              frame 3 {
                n211 = Join Numbers(hi=w450, lo=w449) -> ((hi.lo)=w448:u16)
                n212 = Join Numbers(hi=w447, lo=w446) -> ((hi.lo)=w445:u16)
                n213 = local write "выстрел X LiF 2"(w448) -> ()
                n214 = local write "выстрел Y LiF 2"(w445) -> ()
                "Знак LiF2 Dx" <- w443
              }
              frame 4 {
                n215 = Join Numbers(hi=w458, lo=w457) -> ((hi.lo)=w456:u16)
                n216 = Join Numbers(hi=w455, lo=w454) -> ((hi.lo)=w453:u16)
                n217 = local write "выстрел X Графит"(w456) -> ()
                n218 = local write "выстрел  Y Графит"(w453) -> ()
                "Знак Графит Dx" <- w452
              }
            }
            n219 = case shown="True" "Звук выстрела" {
              tunnel: [w421 w422] -> w409
              tunnel: w408 -> [w421 w422]
              frame False {
              }
              frame True {
                n220 = call <vilib>:"Beep.vi"("use system alert? (T)"=FALSE, "duration (msec)"=u32 400, "frequency (Hz)"=u32 700) -> ()  [unwired: 9 in]
              }
            }
            n221 = property on="XY лазера" class="Bool (strict)"(error in=w409, "Visible"=TRUE) -> (error out=w407:errorcluster)  [unwired: 1 in, 1 out]
            n222 = Increment(x="Выстрел по мишени!") -> (x+1=w414:u32)
            n223 = property on="Выстрел по мишени!" class="DigNum (strict)"(error in=w407, "Val(Sgnl)"=w414) -> (error out=w406:errorcluster)  [unwired: 1 in, 1 out]
          }
          frame 171 {
            # "Текущее положение лазера"
            n224 = case shown="2" w474 {
              tunnel: [w491 w502 w525 w542] -> w463
              tunnel: w473 -> [w483 w497 w514 w531]
              tunnel: w472 -> [w482 w498 w515 w532]
              tunnel: w471 -> [w481 w499 w516 w533]
              tunnel: w470 -> [w480 w500 w517 w534]
              tunnel: w469 -> [w475 w493 w510 w527]
              tunnel: w465 -> [w479 w496 w513 w528]
              frame 1, Default {
                n225 = property on="Знак дейт Dx" class="DigNum (strict)"(error in=w475, "Value"=w479) -> (error out=w476:errorcluster)  [unwired: 1 in, 1 out]
                n226 = Join Numbers(hi=w480, lo=w481) -> ((hi.lo)=w478:u16)
                n227 = Join Numbers(hi=w482, lo=w483) -> ((hi.lo)=w477:u16)
                n228 = local write "выстрел X дейт"(w478) -> ()
                n229 = local write "выстрел Y дейт"(w477) -> ()
                n230 = property on="Дейтерий" class="Pict"(error in=w476) -> (error out=w490:errorcluster, "Position"=w489:T2)  [unwired: 1 in, 1 out]
                n231 = Unbundle(w489) -> ("Left"=w488:i32, "Top"=w487:i32)
                n232 = Add(x=w488, y=w478) -> (x+y=w485:i32)
                n233 = Add(x=w487, y=w477) -> (x+y=w486:i32)
                n234 = Bundle(w485, w486) -> (w484:cluster{i32, i32})  [unwired: 1 in]
                n235 = property on="XY лазера" class="Bool (strict)"(error in=w490, "Position"=w484) -> (error out=w491:errorcluster)  [unwired: 1 in, 1 out]
              }
              frame 2 {
                n236 = property on="Знак LiF1 Dx" class="DigNum (strict)"(error in=w493, "Value"=w496) -> (error out=w492:errorcluster)  [unwired: 1 in, 1 out]
                n237 = Join Numbers(hi=w500, lo=w499) -> ((hi.lo)=w495:u16)
                n238 = Join Numbers(hi=w498, lo=w497) -> ((hi.lo)=w494:u16)
                n239 = local write "выстрел X LiF 1"(w495) -> ()
                n240 = local write "выстрел Y LiF 1"(w494) -> ()
                n241 = property on="LiF 1" class="Pict"(error in=w492) -> (error out=w508:errorcluster, "Position"=w507:T2)  [unwired: 1 in, 1 out]
                n242 = Unbundle(w507) -> ("Left"=w506:i32, "Top"=w501:i32)
                n243 = Add(x=w506, y=w495) -> (x+y=w505:i32)
                n244 = Add(x=w501, y=w494) -> (x+y=w504:i32)
                n245 = Bundle(w505, w504) -> (w503:cluster{i32, i32})  [unwired: 1 in]
                n246 = property on="XY лазера" class="Bool (strict)"(error in=w508, "Position"=w503) -> (error out=w502:errorcluster)  [unwired: 1 in, 1 out]
              }
              frame 3 {
                n247 = property on="Знак LiF2 Dx" class="DigNum (strict)"(error in=w510, "Value"=w513) -> (error out=w509:errorcluster)  [unwired: 1 in, 1 out]
                n248 = Join Numbers(hi=w517, lo=w516) -> ((hi.lo)=w512:u16)
                n249 = Join Numbers(hi=w515, lo=w514) -> ((hi.lo)=w511:u16)
                n250 = local write "выстрел X LiF 2"(w512) -> ()
                n251 = local write "выстрел Y LiF 2"(w511) -> ()
                n252 = property on="LiF 2" class="Pict"(error in=w509) -> (error out=w524:errorcluster, "Position"=w523:T2)  [unwired: 1 in, 1 out]
                n253 = Unbundle(w523) -> ("Left"=w520:i32, "Top"=w519:i32)
                n254 = Add(x=w520, y=w512) -> (x+y=w522:i32)
                n255 = Add(x=w519, y=w511) -> (x+y=w521:i32)
                n256 = Bundle(w522, w521) -> (w518:cluster{i32, i32})  [unwired: 1 in]
                n257 = property on="XY лазера" class="Bool (strict)"(error in=w524, "Position"=w518) -> (error out=w525:errorcluster)  [unwired: 1 in, 1 out]
              }
              frame 4 {
                n258 = property on="Знак Графит Dx" class="DigNum (strict)"(error in=w527, "Value"=w528) -> (error out=w526:errorcluster)  [unwired: 1 in, 1 out]
                n259 = Join Numbers(hi=w534, lo=w533) -> ((hi.lo)=w530:u16)
                n260 = Join Numbers(hi=w532, lo=w531) -> ((hi.lo)=w529:u16)
                n261 = local write "выстрел X Графит"(w530) -> ()
                n262 = local write "выстрел  Y Графит"(w529) -> ()
                n263 = property on="Графит" class="Pict"(error in=w526) -> (error out=w540:errorcluster, "Position"=w539:T2)  [unwired: 1 in, 1 out]
                n264 = Unbundle(w539) -> ("Left"=w538:i32, "Top"=w535:i32)
                n265 = Add(x=w538, y=w530) -> (x+y=w537:i32)
                n266 = Add(x=w535, y=w529) -> (x+y=w536:i32)
                n267 = Bundle(w537, w536) -> (w541:cluster{i32, i32})  [unwired: 1 in]
                n268 = property on="XY лазера" class="Bool (strict)"(error in=w540, "Position"=w541) -> (error out=w542:errorcluster)  [unwired: 1 in, 1 out]
              }
            }
            n269 = property on="XY лазера" class="Bool (strict)"(error in=w463, "Visible"=TRUE) -> (error out=w462:errorcluster)  [unwired: 1 in, 1 out]
            n270 = property on="Статус" class="Bool (strict)"(error in=w462, "Caption.TextColor"=u32 56339 ("цвет")) -> (error out=w467:errorcluster)  [unwired: 1 in, 1 out]
            n271 = property on="Статус" class="Bool (strict)"(error in=w467, "Caption.Text"="Готов!" ("Label.Text")) -> (error out=w459:errorcluster)  [unwired: 1 in, 1 out]
            n272 = property on="Статус" class="Bool (strict)"(error in=w459, "Caption.Position"=T2 {"Left"=970, "Top"=-32}) -> (error out=w461:errorcluster)  [unwired: 1 in, 1 out]
          }
          frame 172 {
            # "Команда занятости"
            n273 = case shown="1, Default" w543 {
              tunnel: [w577 w588 w611 w628] -> w549
              tunnel: w544 -> [w569 w583 w600 w617]
              tunnel: w545 -> [w568 w584 w601 w618]
              tunnel: w546 -> [w567 w585 w602 w619]
              tunnel: w547 -> [w566 w586 w603 w620]
              tunnel: w550 -> [w561 w579 w596 w613]
              tunnel: w548 -> [w565 w582 w599 w614]
              frame 1, Default {
                n274 = property on="Знак дейт Dx" class="DigNum (strict)"(error in=w561, "Value"=w565) -> (error out=w562:errorcluster)  [unwired: 1 in, 1 out]
                n275 = Join Numbers(hi=w566, lo=w567) -> ((hi.lo)=w564:u16)
                n276 = Join Numbers(hi=w568, lo=w569) -> ((hi.lo)=w563:u16)
                n277 = local write "выстрел X дейт"(w564) -> ()
                n278 = local write "выстрел Y дейт"(w563) -> ()
                n279 = property on="Дейтерий" class="Pict"(error in=w562) -> (error out=w576:errorcluster, "Position"=w575:T2)  [unwired: 1 in, 1 out]
                n280 = Unbundle(w575) -> ("Left"=w574:i32, "Top"=w573:i32)
                n281 = Add(x=w574, y=w564) -> (x+y=w571:i32)
                n282 = Add(x=w573, y=w563) -> (x+y=w572:i32)
                n283 = Bundle(w571, w572) -> (w570:cluster{i32, i32})  [unwired: 1 in]
                n284 = property on="XY лазера" class="Bool (strict)"(error in=w576, "Position"=w570) -> (error out=w577:errorcluster)  [unwired: 1 in, 1 out]
              }
              frame 2 {
                n285 = property on="Знак LiF1 Dx" class="DigNum (strict)"(error in=w579, "Value"=w582) -> (error out=w578:errorcluster)  [unwired: 1 in, 1 out]
                n286 = Join Numbers(hi=w586, lo=w585) -> ((hi.lo)=w581:u16)
                n287 = Join Numbers(hi=w584, lo=w583) -> ((hi.lo)=w580:u16)
                n288 = local write "выстрел X LiF 1"(w581) -> ()
                n289 = local write "выстрел Y LiF 1"(w580) -> ()
                n290 = property on="LiF 1" class="Pict"(error in=w578) -> (error out=w594:errorcluster, "Position"=w593:T2)  [unwired: 1 in, 1 out]
                n291 = Unbundle(w593) -> ("Left"=w592:i32, "Top"=w587:i32)
                n292 = Add(x=w592, y=w581) -> (x+y=w591:i32)
                n293 = Add(x=w587, y=w580) -> (x+y=w590:i32)
                n294 = Bundle(w591, w590) -> (w589:cluster{i32, i32})  [unwired: 1 in]
                n295 = property on="XY лазера" class="Bool (strict)"(error in=w594, "Position"=w589) -> (error out=w588:errorcluster)  [unwired: 1 in, 1 out]
              }
              frame 3 {
                n296 = property on="Знак LiF2 Dx" class="DigNum (strict)"(error in=w596, "Value"=w599) -> (error out=w595:errorcluster)  [unwired: 1 in, 1 out]
                n297 = Join Numbers(hi=w603, lo=w602) -> ((hi.lo)=w598:u16)
                n298 = Join Numbers(hi=w601, lo=w600) -> ((hi.lo)=w597:u16)
                n299 = local write "выстрел X LiF 2"(w598) -> ()
                n300 = local write "выстрел Y LiF 2"(w597) -> ()
                n301 = property on="LiF 2" class="Pict"(error in=w595) -> (error out=w610:errorcluster, "Position"=w609:T2)  [unwired: 1 in, 1 out]
                n302 = Unbundle(w609) -> ("Left"=w606:i32, "Top"=w605:i32)
                n303 = Add(x=w606, y=w598) -> (x+y=w608:i32)
                n304 = Add(x=w605, y=w597) -> (x+y=w607:i32)
                n305 = Bundle(w608, w607) -> (w604:cluster{i32, i32})  [unwired: 1 in]
                n306 = property on="XY лазера" class="Bool (strict)"(error in=w610, "Position"=w604) -> (error out=w611:errorcluster)  [unwired: 1 in, 1 out]
              }
              frame 4 {
                n307 = property on="Знак Графит Dx" class="DigNum (strict)"(error in=w613, "Value"=w614) -> (error out=w612:errorcluster)  [unwired: 1 in, 1 out]
                n308 = Join Numbers(hi=w620, lo=w619) -> ((hi.lo)=w616:u16)
                n309 = Join Numbers(hi=w618, lo=w617) -> ((hi.lo)=w615:u16)
                n310 = local write "выстрел X Графит"(w616) -> ()
                n311 = local write "выстрел  Y Графит"(w615) -> ()
                n312 = property on="Графит" class="Pict"(error in=w612) -> (error out=w626:errorcluster, "Position"=w625:T2)  [unwired: 1 in, 1 out]
                n313 = Unbundle(w625) -> ("Left"=w624:i32, "Top"=w621:i32)
                n314 = Add(x=w624, y=w616) -> (x+y=w623:i32)
                n315 = Add(x=w621, y=w615) -> (x+y=w622:i32)
                n316 = Bundle(w623, w622) -> (w627:cluster{i32, i32})  [unwired: 1 in]
                n317 = property on="XY лазера" class="Bool (strict)"(error in=w626, "Position"=w627) -> (error out=w628:errorcluster)  [unwired: 1 in, 1 out]
              }
            }
            n318 = property on="XY лазера" class="Bool (strict)"(error in=w549, "Visible"=FALSE) -> (error out=w555:errorcluster)  [unwired: 1 in, 1 out]
            n319 = property on="Статус" class="Bool (strict)"(error in=w555, "Visible"=TRUE) -> (error out=w556:errorcluster)  [unwired: 1 in, 1 out]
            n320 = property on="Статус" class="Bool (strict)"(error in=w556, "Caption.TextColor"=u32 16711680 ("цвет")) -> (error out=w558:errorcluster)  [unwired: 1 in, 1 out]
            n321 = property on="Статус" class="Bool (strict)"(error in=w558, "Caption.Text"="Идет перемещение..." ("Label.Text")) -> (error out=w551:errorcluster)  [unwired: 1 in, 1 out]
            n322 = property on="Статус" class="Bool (strict)"(error in=w551, "Caption.Position"=T2 {"Left"=800, "Top"=-32}) -> (error out=w552:errorcluster)  [unwired: 1 in, 1 out]
          }
        }
        n323 = Build Array(w209, w208, w207, w206, w205, w204, w203, w202, w201, w200, w199, w198, w197, w195, w194, w193, w192, w191, w190, w196) -> (w211:u16[])
        n324 = Byte Array To String(unsigned byte array=w211) -> (string=w210:string)
        "send string" <- w210
        n325 = TCP Write(connection ID=w189, data in=w210, error in (no error)=w188) -> (error out=w187:errorcluster)  [unwired: 1 in, 2 out]
      }
      event "Выстрел по мишени!": Value Change {
        # "Отрисовка точек на мишенях"
        n326 = event-data() -> ()  [unwired: 7 out]
        n327 = Increment(x="Счетчик выстрелов:") -> (x+1=w635:u32)
        n328 = property on="Счетчик выстрелов:" class="DigNum (strict)"(error in=w633, "Value"=w635) -> (error out=w634:errorcluster)  [unwired: 1 in, 1 out]
        n329 = property on="id мишени" class="DigNum (strict)"(error in=w634) -> (error out=w632:errorcluster, "Value"=w642:u16)  [unwired: 1 in, 1 out]
        n330 = case shown="4" w642 {
          selector: w642 -> [w669 w671 w680 w696 w704]
          tunnel: [_ "Шаг перехода по Х дейт" "Шаг перехода по Х LiF 1" "Шаг перехода по Х LiF 2" "Шаг перехода по Y графит"] -> _
          tunnel: [_ "выстрел Y дейт" "выстрел Y LiF 1" "выстрел Y LiF 2" "выстрел  Y Графит"] -> w636
          tunnel: [_ "Шаг перехода по Y дейт" "Шаг перехода по Y LiF 1" "Шаг перехода по Y LiF 2" "Шаг перехода по Х графит"] -> _
          tunnel: [_ "выстрел X дейт" "выстрел X LiF 1" "выстрел X LiF 2" "выстрел X Графит"] -> w637
          tunnel: [_ "Выстрелов в точку дейтерий" "Выстрелов в точку LiF 1" "Выстрелов в точку  LiF 2" "Выстрелов в точку  графит"] -> _
          tunnel: [_ "Дейтерий" "LiF 1" "LiF 2" "Графит"] -> w643
          tunnel: [_ u32 3381759 ("цвет") u32 16762112 ("цвет") u32 16762112 ("цвет") u32 16448250 ("цвет")] -> w641
          tunnel: [w669 w671 w680 w696 w704] -> w640
          tunnel: w632 -> [w668 w670 w679 w688 w697]
          tunnel: [w668 w670 w679 w688 w697] -> w631
          frame 0, Default {
          }
          frame 1 {
            # "все данный мишени 1 (дейтерий)"
          }
          frame 2 {
            # "все данные мишени 2 (LiF 1)"
          }
          frame 3 {
            # "все данные мишени 3 (LiF 2)"
          }
          frame 4 {
            # "все данные мишени 4 (Графит)"
          }
        }
        n331 = call "Добавить точку на рисунок (SubVI).vi"("in picture"=w643, "dot х"=w637, "dot y"=w636, "thickness"=u16 10, "цвет"=w641, "error in"=w631) -> ("Коорд.X"=w630:u16, "Коорд.Y"=w629:u16, "error out"=w639:errorcluster, "out picture"=w638:picture)  [unwired: 10 in]
        n332 = case shown="4" w640 {
          tunnel: w630 -> [_ w649 w654 w659 w663]
          tunnel: [w647 w652 w657 w662 w667] -> w646
          tunnel: w629 -> [_ w648 w653 w658 w664]
          tunnel: w639 -> [w647 w650 w656 w661 w666]
          tunnel: w638 -> [_ w651 w655 w660 w665]
          frame 0, Default {
          }
          frame 1 {
            n333 = local write "выстрел X дейт"(w649) -> ()
            n334 = property on="Дейтерий" class="Pict"(error in=w650, "Value"=w651) -> (error out=w652:errorcluster)  [unwired: 1 in, 1 out]
            n335 = local write "выстрел Y дейт"(w648) -> ()
          }
          frame 2 {
            n336 = local write "выстрел X LiF 1"(w654) -> ()
            n337 = local write "выстрел Y LiF 1"(w653) -> ()
            n338 = property on="LiF 1" class="Pict"(error in=w656, "Value"=w655) -> (error out=w657:errorcluster)  [unwired: 1 in, 1 out]
          }
          frame 3 {
            n339 = local write "выстрел X LiF 2"(w659) -> ()
            n340 = local write "выстрел Y LiF 2"(w658) -> ()
            n341 = property on="LiF 2" class="Pict"(error in=w661, "Value"=w660) -> (error out=w662:errorcluster)  [unwired: 1 in, 1 out]
          }
          frame 4 {
            n342 = local write "выстрел X Графит"(w663) -> ()
            n343 = local write "выстрел  Y Графит"(w664) -> ()
            n344 = property on="Графит" class="Pict"(error in=w666, "Value"=w665) -> (error out=w667:errorcluster)  [unwired: 1 in, 1 out]
          }
        }
      }
      event "Дейтерий": Shortcut Menu Selection (User) {
        n345 = event-data() -> ("ItemTag"=w707:string)  [unwired: 8 out]
        n346 = case shown="\"Очистить\"" w707 {
          tunnel: w708 -> [w709 w710 w730]
          tunnel: [w709 w711 w729] -> w706
          frame "False", Default {
          }
          frame "Выбрать" {
            n347 = Two Button Dialog(message="Вы уверены, что хотите выбрать эту мишень?", 1:"Нет" ("F button name (\"Cancel\")"), 2:"Да" ("T button name (\"OK\")")) -> (T button?=w712:bool)
            n348 = case shown="True" w712 {
              tunnel: [w716 w721] -> w711
              tunnel: w710 -> [w716 w719]
              frame False {
              }
              frame True {
                w717 = u16 1 ("id мишени")
                n349 = property on="id мишени" class="DigNum (strict)"(error in=w719, "Value"=w717) -> (error out=w718:errorcluster)  [unwired: 1 in, 1 out]
                n350 = property on="id мишени" class="DigNum (strict)"(error in=w718, "Val(Sgnl)"=w717) -> (error out=w720:errorcluster)  [unwired: 1 in, 1 out]
                n351 = property on="Выбор миш 1" class="Bool (strict)"(error in=w720, "Value"=TRUE ("Выбор миш 1")) -> (error out=w728:errorcluster)  [unwired: 1 in, 1 out]
                n352 = property on="Выбор миш 2" class="Bool (strict)"(error in=w728, "Value"=FALSE ("Выбор миш 2")) -> (error out=w727:errorcluster)  [unwired: 1 in, 1 out]
                n353 = property on="Выбор миш 3" class="Bool (strict)"(error in=w727, "Value"=FALSE ("Выбор миш 3")) -> (error out=w726:errorcluster)  [unwired: 1 in, 1 out]
                n354 = property on="Выбор миш 4" class="Bool (strict)"(error in=w726, "Value"=FALSE ("Выбор миш 4")) -> (error out=w721:errorcluster)  [unwired: 1 in, 1 out]
              }
            }
          }
          frame "Очистить" {
            n355 = Two Button Dialog(message="Вы уверены, что хотите очистить эту мишень?", 1:"Нет" ("F button name (\"Cancel\")"), 2:"Да" ("T button name (\"OK\")")) -> (T button?=w731:bool)
            n356 = case shown="True" w731 {
              tunnel: w730 -> [w735 w737]
              tunnel: [w735 w736] -> w729
              frame False {
              }
              frame True {
                n357 = call "Empty Picture"() -> ("empty picture"=w739:picture)
                n358 = local write "Дейтерий"(w739) -> ()
                n359 = property on="id мишени" class="DigNum (strict)"(error in=w737, "Value"=u16 0 ("id мишени")) -> (error out=w736:errorcluster)  [unwired: 1 in, 1 out]
              }
            }
          }
        }
      }
      event "LiF 1": Shortcut Menu Selection (User) {
        # "Очистка мишеней"
        n360 = event-data() -> ("ItemTag"=w740:string)  [unwired: 1 out]
        n361 = case shown="\"Выбрать\"" w740 {
          tunnel: w742 -> [w743 w745 w758]
          tunnel: [w743 w744 w757] -> w741
          frame "False", Default {
          }
          frame "Очистить" {
            n362 = Two Button Dialog(message="Вы уверены, что хотите очистить эту мишень?", 1:"Нет" ("F button name (\"Cancel\")"), 2:"Да" ("T button name (\"OK\")")) -> (T button?=w746:bool)
            n363 = case shown="True" w746 {
              tunnel: w745 -> [w750 w752]
              tunnel: [w750 w752] -> w744
              frame False {
              }
              frame True {
                n364 = call "Empty Picture"() -> ("empty picture"=w751:picture)
                n365 = local write "LiF 1"(w751) -> ()
              }
            }
          }
          frame "Выбрать" {
            n366 = Two Button Dialog(message="Вы уверены, что хотите выбрать эту мишень?", 1:"Нет" ("F button name (\"Cancel\")"), 2:"Да" ("T button name (\"OK\")")) -> (T button?=w753:bool)
            n367 = case shown="True" w753 {
              tunnel: w758 -> [w759 w762]
              tunnel: [w759 w767] -> w757
              frame False {
              }
              frame True {
                w760 = u16 2 ("id мишени")
                n368 = property on="id мишени" class="DigNum (strict)"(error in=w762, "Value"=w760) -> (error out=w761:errorcluster)  [unwired: 1 in, 1 out]
                n369 = property on="id мишени" class="DigNum (strict)"(error in=w761, "Val(Sgnl)"=w760) -> (error out=w771:errorcluster)  [unwired: 1 in, 1 out]
                n370 = property on="Выбор миш 1" class="Bool (strict)"(error in=w771, "Value"=FALSE ("Выбор миш 1")) -> (error out=w770:errorcluster)  [unwired: 1 in, 1 out]
                n371 = property on="Выбор миш 2" class="Bool (strict)"(error in=w770, "Value"=TRUE ("Выбор миш 2")) -> (error out=w769:errorcluster)  [unwired: 1 in, 1 out]
                n372 = property on="Выбор миш 3" class="Bool (strict)"(error in=w769, "Value"=FALSE ("Выбор миш 3")) -> (error out=w768:errorcluster)  [unwired: 1 in, 1 out]
                n373 = property on="Выбор миш 4" class="Bool (strict)"(error in=w768, "Value"=FALSE ("Выбор миш 4")) -> (error out=w767:errorcluster)  [unwired: 1 in, 1 out]
              }
            }
          }
        }
      }
      event "LiF 2": Shortcut Menu Selection (User) {
        # "Очистка мишеней"
        n374 = event-data() -> ("ItemTag"=w772:string)  [unwired: 8 out]
        n375 = case shown="\"Выбрать\"" w772 {
          tunnel: w774 -> [w775 w777 w786]
          tunnel: [w775 w776 w785] -> w773
          frame "False", Default {
          }
          frame "Очистить" {
            n376 = Two Button Dialog(message="Вы уверены, что хотите очистить эту мишень?", 1:"Нет" ("F button name (\"Cancel\")"), 2:"Да" ("T button name (\"OK\")")) -> (T button?=w778:bool)
            n377 = case shown="True" w778 {
              tunnel: w777 -> [w782 w784]
              tunnel: [w782 w784] -> w776
              frame False {
              }
              frame True {
                n378 = call "Empty Picture"() -> ("empty picture"=w783:picture)
                n379 = local write "LiF 2"(w783) -> ()
              }
            }
          }
          frame "Выбрать" {
            n380 = Two Button Dialog(message="Вы уверены, что хотите выбрать эту мишень?", 1:"Нет" ("F button name (\"Cancel\")"), 2:"Да" ("T button name (\"OK\")")) -> (T button?=w787:bool)
            n381 = case shown="True" w787 {
              tunnel: [w791 w796] -> w785
              tunnel: w786 -> [w791 w794]
              frame False {
              }
              frame True {
                w792 = u16 3 ("id мишени")
                n382 = property on="id мишени" class="DigNum (strict)"(error in=w794, "Value"=w792) -> (error out=w793:errorcluster)  [unwired: 1 in, 1 out]
                n383 = property on="id мишени" class="DigNum (strict)"(error in=w793, "Val(Sgnl)"=w792) -> (error out=w795:errorcluster)  [unwired: 1 in, 1 out]
                n384 = property on="Выбор миш 1" class="Bool (strict)"(error in=w795, "Value"=FALSE ("Выбор миш 1")) -> (error out=w803:errorcluster)  [unwired: 1 in, 1 out]
                n385 = property on="Выбор миш 2" class="Bool (strict)"(error in=w803, "Value"=FALSE ("Выбор миш 2")) -> (error out=w802:errorcluster)  [unwired: 1 in, 1 out]
                n386 = property on="Выбор миш 3" class="Bool (strict)"(error in=w802, "Value"=TRUE ("Выбор миш 3")) -> (error out=w801:errorcluster)  [unwired: 1 in, 1 out]
                n387 = property on="Выбор миш 4" class="Bool (strict)"(error in=w801, "Value"=FALSE ("Выбор миш 4")) -> (error out=w796:errorcluster)  [unwired: 1 in, 1 out]
              }
            }
          }
        }
      }
      event "Графит": Shortcut Menu Selection (User) {
        # "Очистка мишеней"
        n388 = event-data() -> ("ItemTag"=w804:string)  [unwired: 8 out]
        n389 = case shown="\"Выбрать\"" w804 {
          tunnel: w806 -> [w807 w809 w818]
          tunnel: [w807 w808 w817] -> w805
          frame "False", Default {
          }
          frame "Очистить" {
            n390 = Two Button Dialog(message="Вы уверены, что хотите очистить эту мишень?", 1:"Нет" ("F button name (\"Cancel\")"), 2:"Да" ("T button name (\"OK\")")) -> (T button?=w810:bool)
            n391 = case shown="True" w810 {
              tunnel: w809 -> [w814 w816]
              tunnel: [w814 w816] -> w808
              frame False {
              }
              frame True {
                n392 = call "Empty Picture"() -> ("empty picture"=w815:picture)
                n393 = local write "Графит"(w815) -> ()
              }
            }
          }
          frame "Выбрать" {
            n394 = Two Button Dialog(message="Вы уверены, что хотите выбрать эту мишень?", 1:"Нет" ("F button name (\"Cancel\")"), 2:"Да" ("T button name (\"OK\")")) -> (T button?=w819:bool)
            n395 = case shown="True" w819 {
              tunnel: [w823 w824] -> w817
              tunnel: w818 -> [w823 w837]
              frame False {
              }
              frame True {
                w835 = u16 4 ("id мишени")
                n396 = property on="id мишени" class="DigNum (strict)"(error in=w837, "Value"=w835) -> (error out=w836:errorcluster)  [unwired: 1 in, 1 out]
                n397 = property on="id мишени" class="DigNum (strict)"(error in=w836, "Val(Sgnl)"=w835) -> (error out=w838:errorcluster)  [unwired: 1 in, 1 out]
                n398 = property on="Выбор миш 1" class="Bool (strict)"(error in=w838, "Value"=FALSE ("Выбор миш 1")) -> (error out=w845:errorcluster)  [unwired: 1 in, 1 out]
                n399 = property on="Выбор миш 2" class="Bool (strict)"(error in=w845, "Value"=FALSE ("Выбор миш 2")) -> (error out=w844:errorcluster)  [unwired: 1 in, 1 out]
                n400 = property on="Выбор миш 3" class="Bool (strict)"(error in=w844, "Value"=FALSE ("Выбор миш 3")) -> (error out=w843:errorcluster)  [unwired: 1 in, 1 out]
                n401 = property on="Выбор миш 4" class="Bool (strict)"(error in=w843, "Value"=TRUE ("Выбор миш 4")) -> (error out=w825:errorcluster)  [unwired: 1 in, 1 out]
                n402 = property on="Графит" class="Pict"(error in=w825) -> (error out=w832:errorcluster, "Position"=w831:T2)  [unwired: 1 in, 1 out]
                n403 = local read "выстрел  Y Графит"() -> (w834:u16)
                n404 = local read "выстрел X Графит"() -> (w833:u16)
                n405 = Unbundle(w831) -> ("Left"=w829:i32, "Top"=w826:i32)
                n406 = Add(x=w829, y=w833) -> (x+y=w828:i32)
                n407 = Add(x=w826, y=w834) -> (x+y=w827:i32)
                n408 = Bundle(w828, w827) -> (w830:cluster{i32, i32})  [unwired: 1 in]
                n409 = property on="XY лазера" class="Bool (strict)"(error in=w832, "Position"=w830) -> (error out=w824:errorcluster)  [unwired: 1 in, 1 out]
              }
            }
          }
        }
      }
      event Mouse Move {
        # "Работа с курсором - линейка"
        n410 = event-data() -> ()  [unwired: 6 out]
        n411 = control-ref of="This VI"() -> (w871:refnum<vi>)
        n412 = property class="VI"(reference=w871, error in=w847) -> (error out=w846:errorcluster, "Front Panel.PanelBounds"=w870:T5)  [unwired: 1 out]
        n413 = Unbundle By Name(w870) -> ("Left"=w869:i16, "Top"=w868:i16)
        n414 = call-poly <vilib>:"Acquire Input Data.vi"("device ID"=w874, "error in (no error)"=w846) -> ("device ID"=w873:refnum<k1>, "axis info"=w872:T6, "error out"=w867:errorcluster)  [unwired: 1 in, 14 out]
        n415 = Unbundle By Name(w872) -> ("Horizontal"=w865:i32, "Vertical"=w863:i32)
        n416 = To Unsigned Long Integer(number=w869) -> (unsigned 32bit integer=w866:u32)
        n417 = To Unsigned Long Integer(number=w868) -> (unsigned 32bit integer=w864:u32)
        n418 = Subtract(x=w865, y=w866) -> (x-y=w862:u32)
        n419 = Subtract(x=w863, y=w864) -> (x-y=w861:u32)
        n420 = expression code="(x-50)/10" "сдвигаем 0 коорд. по X и приводим к мм"(w862) -> (w856:u32)
        n421 = expression code="(x-47)/10" "сдвигаем 0 коорд. по Y и приводим к мм"(w861) -> (w855:u32)
        n422 = Greater?(x=w855, y=60) -> (0:w853:bool)
        n423 = Greater?(x=w856, y=100) -> (0:w852:bool)
        n424 = Or(x=w852, y=w853) -> (x .or. y?=w854:bool)
        n425 = Select(t=0, s=w854, f=w855) -> (s? t:f=w849:u32)
        "Mouse on Pane pos Vertical" <- w849
        "Slide Y axis" <- w849
        n426 = Equal To 0?(x=w849) -> (x = 0?=w851:bool)
        n427 = Compound Arithmetic op=OR(w853, w852, w851) -> (w850:bool)
        n428 = Select(t=0, s=w850, f=w856) -> (s? t:f=→"Mouse on Pane pos Horizontal" →"Slide X axis":u32)
      }
      event "OK Button": Value Change {
        n429 = event-data() -> ("OldVal"=w875:bool)  [unwired: 2 out]
        n430 = property on="OK Button" class="Bool (strict)"(error in=w877, "Value"=w875) -> (error out=w876:errorcluster)  [unwired: 1 in, 1 out]
        n431 = property on="Счетчик мишеней" class="DigNum (strict)"(error in=w876) -> (error out=w879:errorcluster, "Value"=w881:u16)  [unwired: 1 in, 1 out]
        n432 = Increment(x=w881) -> (x+1=w880:u16)
        "Счетчик мишеней" <- w880
        n433 = case shown="0, Default" w880 {
          tunnel: w879 -> [w882 w887 w891]
          tunnel: [w882 w884 w888] -> w878
          frame 0, Default {
          }
          frame 1 {
            n434 = property on="Мишень 1" class="Pict"(error in=w887, "Visible"=TRUE) -> (error out=w885:errorcluster)  [unwired: 1 in, 1 out]
            n435 = property on="Мишень 2" class="Pict"(error in=w885, "Visible"=FALSE) -> (error out=w884:errorcluster)  [unwired: 1 in, 1 out]
          }
          frame 2 {
            n436 = property on="Мишень 1" class="Pict"(error in=w891, "Visible"=TRUE) -> (error out=w889:errorcluster)  [unwired: 1 in, 1 out]
            n437 = property on="Мишень 2" class="Pict"(error in=w889, "Visible"=TRUE) -> (error out=w888:errorcluster)  [unwired: 1 in, 1 out]
          }
        }
      }
      event "Мишень 1": Shortcut Menu Selection (User) {
        n438 = event-data() -> ("ItemTag"=w895:string)  [unwired: 1 out]
        n439 = case shown="\"Настроить\", Default" w895 {
          tunnel: w894 -> [w899 w911 w912]
          tunnel: [w896 w911 w912] -> w893
          frame "Настроить", Default {
            n440 = call "Настройки мишени (Sub VI).vi"("Параметры мишеней вх"="Параметры М1", "error in"=w899) -> ("Параметры мишеней вых"=w898:T7, "error out"=w897:errorcluster)  [unwired: 16 in]
            n441 = property on="Параметры М1" class="Clust (strict)"(error in=w897, "Value"=w898) -> (error out=w896:errorcluster)  [unwired: 1 in, 1 out]
            n442 = Unbundle(w898) -> ("Название мишени"=w910:string, "Х0"=w909:u16, "Y0"=w908:u16, "Длина, мм"=w906:u16, "Ширина, мм"=w905:u16, "Шаг перехода по горизонтали"=→"Шаг перехода по горизонтали":u16, "Шаг перехода по вертикали"=→"Шаг перехода по вертикали":u16, "Выстрелов до перехода"=→"Выстрелов до перехода":u16)
            n443 = property on="Мишень 1" class="Pict"("TipStrip"=w910) -> ()  [unwired: 2 in, 2 out]
            n444 = Bundle("Х0"=w909, "Y0"=w908) -> (w901:cluster{"Х0":u16, "Y0":u16})  [unwired: 1 in]
            n445 = Bundle("Длина, мм"=w906, "Ширина, мм"=w905) -> (w907:cluster{"Длина, мм":u16, "Ширина, мм":u16})  [unwired: 1 in]
            n446 = property on="Мишень 1" class="Pict"("Position"=w901) -> ()  [unwired: 2 in, 2 out]
            n447 = property on="Мишень 1" class="Pict"("Draw Area Size"=w907) -> ()  [unwired: 2 in, 2 out]
          }
          frame "Выбрать" {
          }
          frame "Очистить" {
          }
        }
      }
      event "id мишени", "Выстрелов в точку дейтерий", "Выстрелов в точку LiF 1", "Выстрелов в точку  LiF 2", "Выстрелов в точку  графит", "Шаг перехода по Х дейт", "Шаг перехода по Х LiF 1", "Шаг перехода по Х LiF 2", "Шаг перехода по Х графит", "Шаг перехода по Y дейт", "Шаг перехода по Y LiF 1", "Шаг перехода по Y LiF 2", "Шаг перехода по Y графит", "Выстрелов до перемотки": Value Change {
        w916 = u8 0 ("element")
        # "обновление информации по мишеням"
        n448 = event-data() -> ()  [unwired: 5 out]
        n449 = property on="Выстрелов до перемотки" class="DigNum (strict)"() -> ("Value"=w917:u16)  [unwired: 2 in, 2 out]
        n450 = local read "id мишени"() -> (w913:u16)
        n451 = Split Number(x=w917) -> (hi(x)=w915:u8, lo(x)=w914:u8)
        n452 = Build Array(u8 85 ("element"), w913, w915, w914, w916, w916, w916, w916, w916, w916, w916, w916, w916, w916, w916, w916, w916, w916, w916, w916) -> (w923:u16[])
        n453 = property on="TCP con ID" class="Ref (strict)"(error in=w919) -> (error out=w922:errorcluster, "Value"=w921:refnum<k5>)  [unwired: 1 in, 1 out]
        n454 = Byte Array To String(unsigned byte array=w923) -> (string=w920:string)
        "on event" <- w920
        n455 = TCP Write(connection ID=w921, data in=w920, error in (no error)=w922) -> (error out=w918:errorcluster)  [unwired: 1 in, 2 out]
      }
      event Panel Close? {
        # "Защита и сохранение при закрытии программы"
        n456 = event-data() -> ()  [unwired: 5 out]
        n457 = Two Button Dialog(message="Вы уверены, что хотите закрыть программу?", 1:"Нет" ("F button name (\"Cancel\")"), 2:"Да" ("T button name (\"OK\")")) -> (T button?=w927:bool)
        n458 = Not(x=w927) -> (.not. x?=w926:bool)
        n459 = case shown="False" w926 {
          selector: w926 -> [w931 w953]
          tunnel: [w934 w953] -> w925
          frame False {
            n460 = flat-sequence {
              tunnel: [w938] -> w936
              tunnel: [w937] -> w932
              tunnel: w931 -> [w937]
              tunnel: w936 -> [w942]
              tunnel: [w942] -> w935
              tunnel: [w940] -> w933
              tunnel: w932 -> [w940]
              tunnel: w935 -> [w947]
              tunnel: [w944] -> w934
              tunnel: w933 -> [w944]
              frame #0 {
                n461 = local read "TCP con ID"() -> (w939:refnum<k5>)
                n462 = TCP Close Connection(connection ID=w939) -> (error out=w938:errorcluster)  [unwired: 1 in, 2 out]
              }
              frame #1 {
                n463 = Wait (ms)(milliseconds to wait=u32 200) -> ()  [unwired: 1 out]
              }
              frame #2 {
                w949 = FALSE ("Запись в файл")
                w948 = TRUE ("Tool Bar:Visible")
                n464 = disable-structure shown="Enabled" {
                  disable-tunnel: [w951 w952] -> w945
                  disable-tunnel: w947 -> [w950 w952]
                  frame Disabled {
                    n465 = Close File(error in=w950) -> (error out=w951:errorcluster)  [unwired: 1 in, 1 out]
                  }
                  frame Enabled {
                  }
                }
                n466 = local write "Connected"(w949) -> ()
                n467 = local write "Con"(w949) -> ()
                n468 = property on="кнопки запуска, стоп и тд" class="VI"(error in=w945, "TB.Visible"=w948) -> (error out=w946:errorcluster)  [unwired: 1 in, 1 out]
                n469 = local write "con err"(w948) -> ()
                n470 = call <vilib>:"General Error Handler.vi"("type of dialog (OK msg:1)"=u32 0 ("milliseconds to wait"), "error in (no error)"=w946) -> ()  [unwired: 14 out]
              }
            }
          }
          frame True {
          }
        }
        n471 = event-data("Discard?"=w925) -> ()  [unwired: 1 in, 1 out]
      }
    }
    n472 = call <vilib>:"General Error Handler.vi"("type of dialog (OK msg:1)"=u8 0, "error in (no error)"=w161) -> ("error out"=w160:errorcluster)  [unwired: 13 out]
  }
  n473 = property class="VI"(error in=w42, "Front Panel.Resizeable"=FALSE ("Front Panel Window:Resizable")) -> (error out=w41:errorcluster)  [unwired: 1 in, 1 out]
  n474 = property on="Выбор миш 1" class="Bool (strict)"(error in=w24, "Value"=TRUE ("Выбор миш 1")) -> (error out=w25:errorcluster)  [unwired: 1 in, 1 out]
  n475 = property class="VI"(error in=w41, "Front Panel.ShowMenuBar"=FALSE ("Front Panel Window:Show Menu Bar")) -> ()  [unwired: 1 in, 2 out]
  n476 = property on="Выбор миш 2" class="Bool (strict)"(error in=w25, "Value"=FALSE ("Выбор миш 2")) -> (error out=w26:errorcluster)  [unwired: 1 in, 1 out]
  n477 = property on="Выбор миш 3" class="Bool (strict)"(error in=w26, "Value"=FALSE ("Выбор миш 3")) -> (error out=w27:errorcluster)  [unwired: 1 in, 1 out]
  n478 = property on="Выбор миш 4" class="Bool (strict)"(error in=w27, "Value"=FALSE ("Выбор миш 4")) -> ()  [unwired: 1 in, 2 out]
  n479 = call-poly <vilib>:"Close Input Device.vi"("error in (no error)"=w1) -> ()  [unwired: 1 in, 9 out]
